vi "gums_measureLoopV3.vi"(0 "File Name":path=path "D:/users/test.dat", 1 "SaveDataQuery":bool=TRUE, 2 "Gain Cluster 2":T4={"Vsd"="Gate", "I 2probe 2"="Gate", "Vxy"="Gate", "Vxx"="Gate", "I leak BG"="Gate", "I leak TG"="Gate", "I Gain 1"=1000000.0, "V Gain 1"=1.0, "conversion factor BG"=1.0, "Vin / Vout 1"=1.0, "V Gain 2"=1.0, "Vin / Vout 2"=1.0, "V Gain 3"=1.0, "Vin / Vout 3"=1.0, "I Gain 2"=1000000.0, "I Gain 3"=1000000.0, "V BG"="Gate", "V TG"="Gate", "conversion factor TG"=1.0, "Vin / Vout 4"=1.0, "Vin / Vout 5"=1.0, "Manual Gain 1"=1.0, "Manual Gain 2"=1.0, "Manual Gain 3"=1.0, "V / I 4"="Gate", "V / I 3"="Gate", "Gain V/I3"=1.0, "Gain V/I4"=1.0} {"conversion factor TG" items=["1 V/V"=1.0, "4 V/V"=4.0, "15 V/V"=15.0, "30 V/V"=30.0, "45 V/V"=45.0]; "I Gain 3" items=["1"=1.0, "10"=10.0, "100"=100.0, "1K"=1000.0, "10K"=10000.0, "100K"=100000.0, "1M"=1000000.0, "10M"=10000000.0, "100M"=100000000.0, "1G"=1000000000.0]; "I Gain 2" items=["1"=1.0, "10"=10.0, "100"=100.0, "1K"=1000.0, "10K"=10000.0, "100K"=100000.0, "1M"=1000000.0, "10M"=10000000.0, "100M"=100000000.0, "1G"=1000000000.0]; "V Gain 3" items=["1"=1.0, "10"=10.0, "100"=100.0, "1K"=1000.0, "10K"=10000.0]; "V Gain 2" items=["1"=1.0, "10"=10.0, "100"=100.0, "1K"=1000.0, "10K"=10000.0]; "conversion factor BG" items=["1 V/V"=1.0, "4 V/V"=4.0, "15 V/V"=15.0, "30 V/V"=30.0, "45 V/V"=45.0]; "V Gain 1" items=["1"=1.0, "10"=10.0, "100"=100.0, "1K"=1000.0, "10K"=10000.0]; "I Gain 1" items=["1"=1.0, "10"=10.0, "100"=100.0, "1K"=1000.0, "10K"=10000.0, "100K"=100000.0, "1M"=1000000.0, "10M"=10000000.0, "100M"=100000000.0, "1G"=1000000000.0]}, 3 "Refresh Rate [ms]":i32=1000 min=0, 4 "Device Cluster":T5={"K2400 1"="", "K2400_1"=FALSE, "K2400 2"="", "K2400_2"=FALSE, "TIC"="", "Tcontrol"="OFF", "DAC"="", "DAC present"=FALSE, "Bfield query"=FALSE, "Wvlen query"=FALSE, "ITC signal"={"ITC"=0, "Signal"=enum."Sensor 1"}, "DMMX"=[["DMM1", ""]], "LockinX"=[["DMM1", ""]]}) -> ()   [LabVIEW 2011]
uses:
  Kelvinox drivers/ITCAPPS - Copie.LLB/ITCSignal.ctl
  Kelvinox drivers/ITCAPPS.LLB/ITCSignals.ctl
  Kelvinox drivers/BUSGEN.LLB/OxfordAddress.ctl
  stopButton.vi
  DAC/DACreadglobal.vi
  GlobalVar.vi
  monochromatorcontrol/perHandlemonochromator.vi
  Tglobalvar.vi
  monochromatorcontrol/libPhyspec.lvlib
panel:
  out "*(type *) &x":refnum<visa-resource-name>
  out "V/I4 array":dbl[](array[numeric])
  out "V/I3 array":dbl[](array[numeric])
  out "SetInstrument Cluster":cluster{dbl, dbl, dbl, dbl[], dbl, dbl, dbl}
  out "Lockin A all (V)":dbl[](array[numeric])
  out "Lockin A Array":dbl[][](array[numeric])
  out "signal cluster":T1
  out "Lockin Y all (V)":dbl[](array[numeric])
  out "Lockin X all (V)":dbl[](array[numeric])
  out "Lockin Y Array":dbl[][](array[numeric])
  out "Lockin X Array":dbl[][](array[numeric])
  out "LockinX":string[][](array[string])
  out "refnum raw":refnum<file>
  out "DMM all (V)":dbl[](array[numeric])
  out "DMM Array":dbl[][](array[numeric])
  out "DMMX":string[][](array[string])
  out "DAC 2 V [V]":dbl=1916.0
  out "DAC 2 array":dbl[](array[numeric])
  out "Formula4Array":dbl[](array[numeric]) format="%.2f"
  out "Formula3Array":dbl[](array[numeric]) format="%.2f"
  out "Formula2Array":dbl[](array[numeric]) format="%.2f"
  in  "Formula 4":string
  in  "Formula 3":string
  in  "Formula 2":string
  out "Formula1Array":dbl[](array[numeric]) format="%.2f"
  in  "Formula 1":string
  out "Rxy Array":dbl[](array[numeric])
  out "ITC signal":T2={"ITC"=0, "Signal"=enum."Sensor 1"}
  in  "Fig4 Y scale":string(combo)="0"
  in  "Y-Axis 4":string(combo)="Gate"
  in  "X-Axis 4":string(combo)="Gate"
  out "Isd 4":cluster{"Bg":dbl[], "V_4probe":dbl[]}(graph)
  in  "Fig3 Y scale":string(combo)="0"
  in  "Y-Axis 3":string(combo)="Gate"
  in  "X-Axis 3":string(combo)="Gate"
  in  "Fig1 Y scale":string(combo)="0"
  in  "Fig2 Y scale":string(combo)="0"
  out "Fig 2":cluster{"Bg":dbl[], "V_4probe":dbl[]}(graph)
  in  "Y-Axis 1":string(combo)="Gate"
  in  "X-Axis 1":string(combo)="Gate"
  out "R4probe array":dbl[](array[numeric])
  out "R2probe array":dbl[](array[numeric])
  out "Itg array":dbl[](array[numeric])
  out "Ibg array":dbl[](array[numeric])
  out "Vxy array":dbl[](array[numeric])
  out "Vxx array":dbl[](array[numeric])
  out "Isd array":dbl[](array[numeric])
  out "Vsd array":dbl[](array[numeric])
  out "Vtg array":dbl[](array[numeric])
  out "Vbg array":dbl[](array[numeric])
  out "R 4probe [kOhm]":dbl=1916.0
  out "V_topgate [V]":dbl=1916.0
  out "V_backgate [V]":dbl=1916.0
  out "Vxy [V]":dbl=1916.0
  out "Vxx [V]":dbl=1916.0
  out "R 2probe [kOhm]":dbl=1916.0
  out "I Leak TG[nA]":dbl=1916.0
  out "I Leak BG [nA]":dbl=1916.0
  out "I 2probe [nA]":dbl=1916.0
  out "Vsd [V]":dbl=1916.0
  in  "Sensitivity Lockin2":T6(ring)
  in  "Sensitivity Lockin1":T6(ring)
  out "Wavelength array":dbl[](array[numeric])
  out "Wavelength [nm]":dbl=1916.0
  out "Wvlen query":bool
  out "refnum data":refnum<file>
  in  "Y-Axis 2":string(combo)="Gate"
  in  "X-Axis 2":string(combo)="Gate"
  out "I K2400 01":dbl[](array[numeric])
  out "I K2400 02":dbl[](array[numeric])
  out "DAC 4 array":dbl[](array[numeric])
  out "DAC 3 array":dbl[](array[numeric])
  out "B":dbl[](array[numeric])
  out "B [T]":dbl=1916.0
  out "T [K]":dbl=1916.0
  out "Bfield query":bool
  out "I K2400_2 [A]":dbl=1916.0
  out "V / I 4 [V or A]":dbl=1916.0
  out "V / I 3 [V or A]":dbl=1916.0
  out "DAC 4 V [V]":dbl=1916.0
  out "DAC 3 V [V]":dbl=1916.0
  out "I K2400_1 [A]":dbl=1916.0
  out "Lockin1 Y [V]":dbl=1916.0
  out "Lockin1 X [V]":dbl=1916.0
  out "Lockin1 Ampl [V]":dbl=1916.0
  out "K2400 1 [V]":dbl=1916.0
  out "K2400 2 [V]":dbl=1916.0
  out "DAC 1 V [V]":dbl=1916.0
  out "DAC present":bool
  out "K2400_2":bool
  out "K2400 2":refnum<visa-resource-name>="GPIB0::11::INSTR"
  out "DAC":refnum<visa-resource-name>="GPIB0::11::INSTR"
  out "Tcontrol":string
  out "K2400_1":bool
  out "TIC":refnum<visa-resource-name>="GPIB0::11::INSTR"
  out "K2400 1":refnum<visa-resource-name>="GPIB0::11::INSTR"
  out "Isd":cluster{"Bg":dbl[], "V_4probe":dbl[]}(graph)
  out "Isd 3":cluster{"Bg":dbl[], "V_4probe":dbl[]}(graph)
  out "stopMainLoop":bool
  out "V K2400_01 array":dbl[](array[numeric])
  out "DAC 1 array":dbl[](array[numeric])
  out "V K2400_02 array":dbl[](array[numeric])
  out "T":dbl[](array[numeric])
  out "Time":dbl[](array[numeric])
  out "Time [s]":dbl=1916.0
  in  "stop":bool
  # "Current run values"
  # "Magnetic Field"
  # "Wavelength"
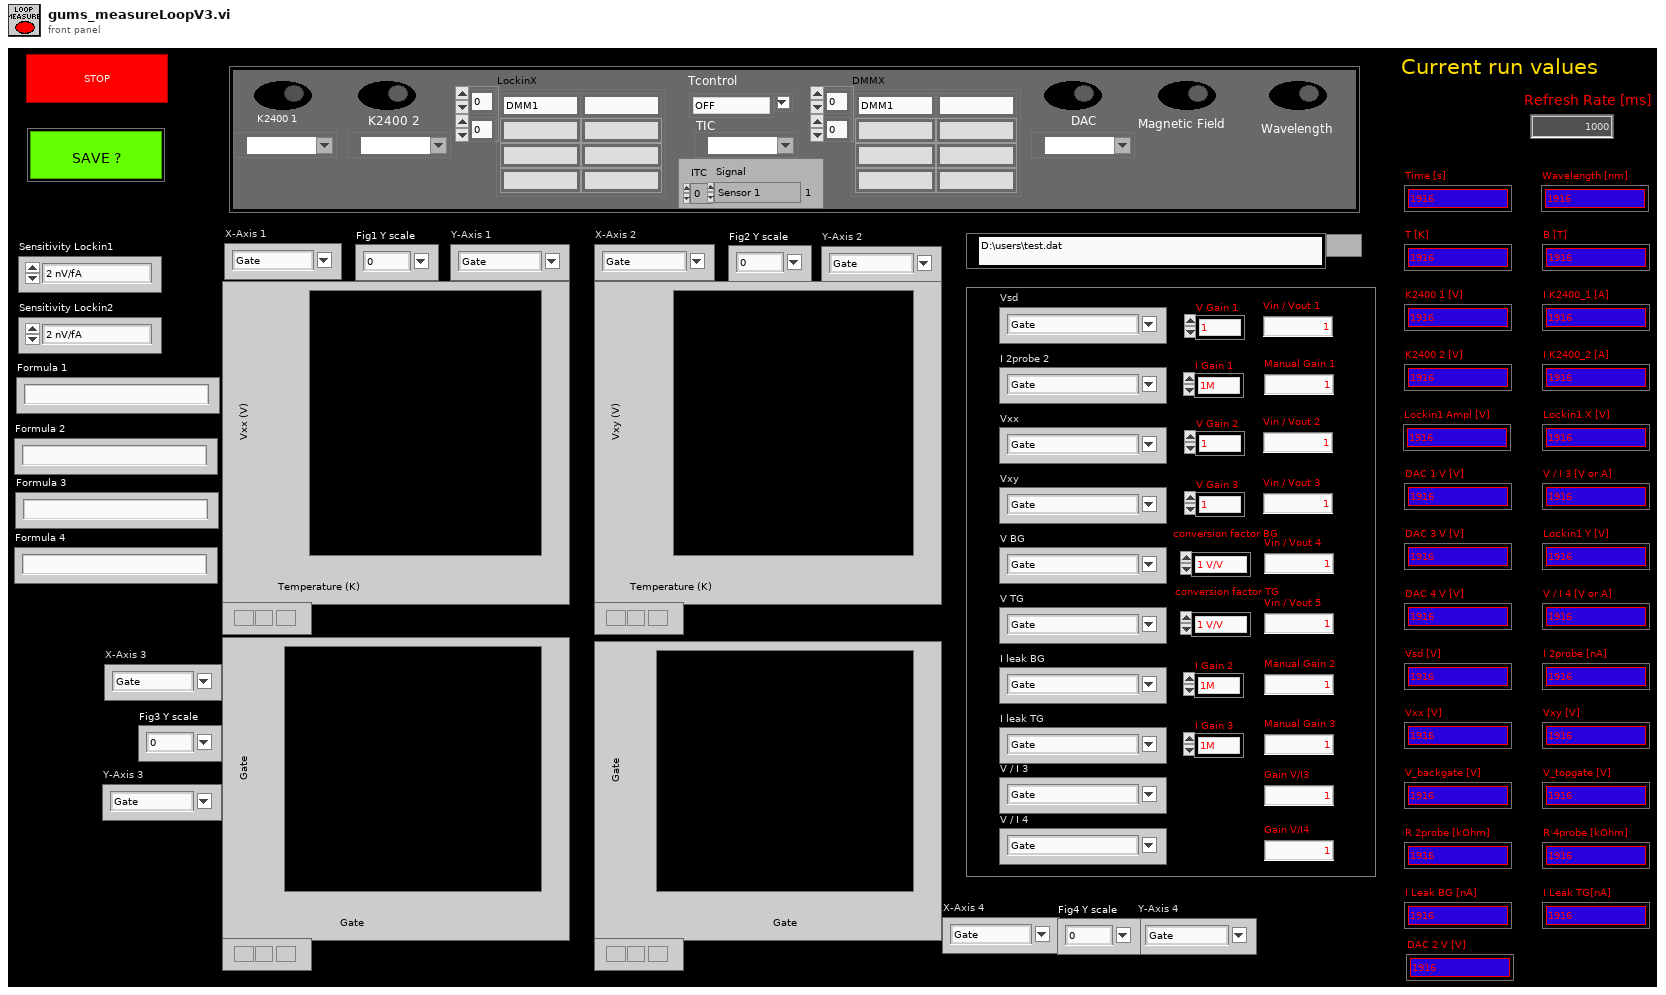
[diagram p1: front panel]
types:
  T1 = cluster{dbl[], dbl[], "I K2400_1 [A]":dbl, "I K2400_2 [A]":dbl, dbl[]}
  T2 = typedef "ITCSignal.ctl" = cluster{"ITC":u16, "Signal":T3}
  T3 = typedef "ITCSignals.ctl" = enum16{"Setpoint", "Sensor 1", "Sensor 2", "Sensor 3", "Needle Valve %", "Heater %"}
  T4 = cluster{"Vsd":string, "I 2probe 2":string, "Vxy":string, "Vxx":string, "I leak BG":string, "I leak TG":string, "I Gain 1":dbl, "V Gain 1":dbl, "conversion factor BG":dbl, "Vin / Vout 1":dbl, "V Gain 2":dbl, "Vin / Vout 2":dbl, "V Gain 3":dbl, "Vin / Vout 3":dbl, "I Gain 2":dbl, "I Gain 3":dbl, "V BG":string, "V TG":string, "conversion factor TG":dbl, "Vin / Vout 4":dbl, "Vin / Vout 5":dbl, "Manual Gain 1":dbl, "Manual Gain 2":dbl, "Manual Gain 3":dbl, "V / I 4":string, "V / I 3":string, "Gain V/I3":dbl, "Gain V/I4":dbl}
  T5 = cluster{"K2400 1":refnum<visa-resource-name>, "K2400_1":bool, "K2400 2":refnum<visa-resource-name>, "K2400_2":bool, "TIC":refnum<visa-resource-name>, "Tcontrol":string, "DAC":refnum<visa-resource-name>, "DAC present":bool, "Bfield query":bool, "Wvlen query":bool, "ITC signal":T2, "DMMX":string[][], "LockinX":string[][]}
  T6 = enum16{"2 nV/fA", "5 nV/fA", "10 nV/fA", "20 nV/fA", "50 nV/fA", "100 nV/fA", "200 nV/fA", "500 nV/fA", "1 uV/pA", "2 uV/pA", "5 uV/pA", "10 uV/pA", "20 uV/pA", "50 uV/pA", "100 uV/pA", "200 uV/pA", "500 uV/pA", "1 mV/nA", "2 mV/nA", "5 mV/nA", "10 mV/nA", "20 mV/nA", "50 mV/nA", "100 mV/nA", "200 mV/nA", "500 mV/nA", "1 V/uA"}
  T7 = typedef "OxfordAddress.ctl" = cluster{"Com Port":i32, "ISOBUS Address":i32, "GPIB Address":i16, "Communication":enum16{"RS232", "ISOBUS", "GPIB", "Gateway"}}
  T8 = enum16{"open", "replace", "create", "open or create", "replace or create", "replace or create with confirmation"}
  T9 = cluster{"Formula4Array":dbl[], "Formula4Array":dbl[]}
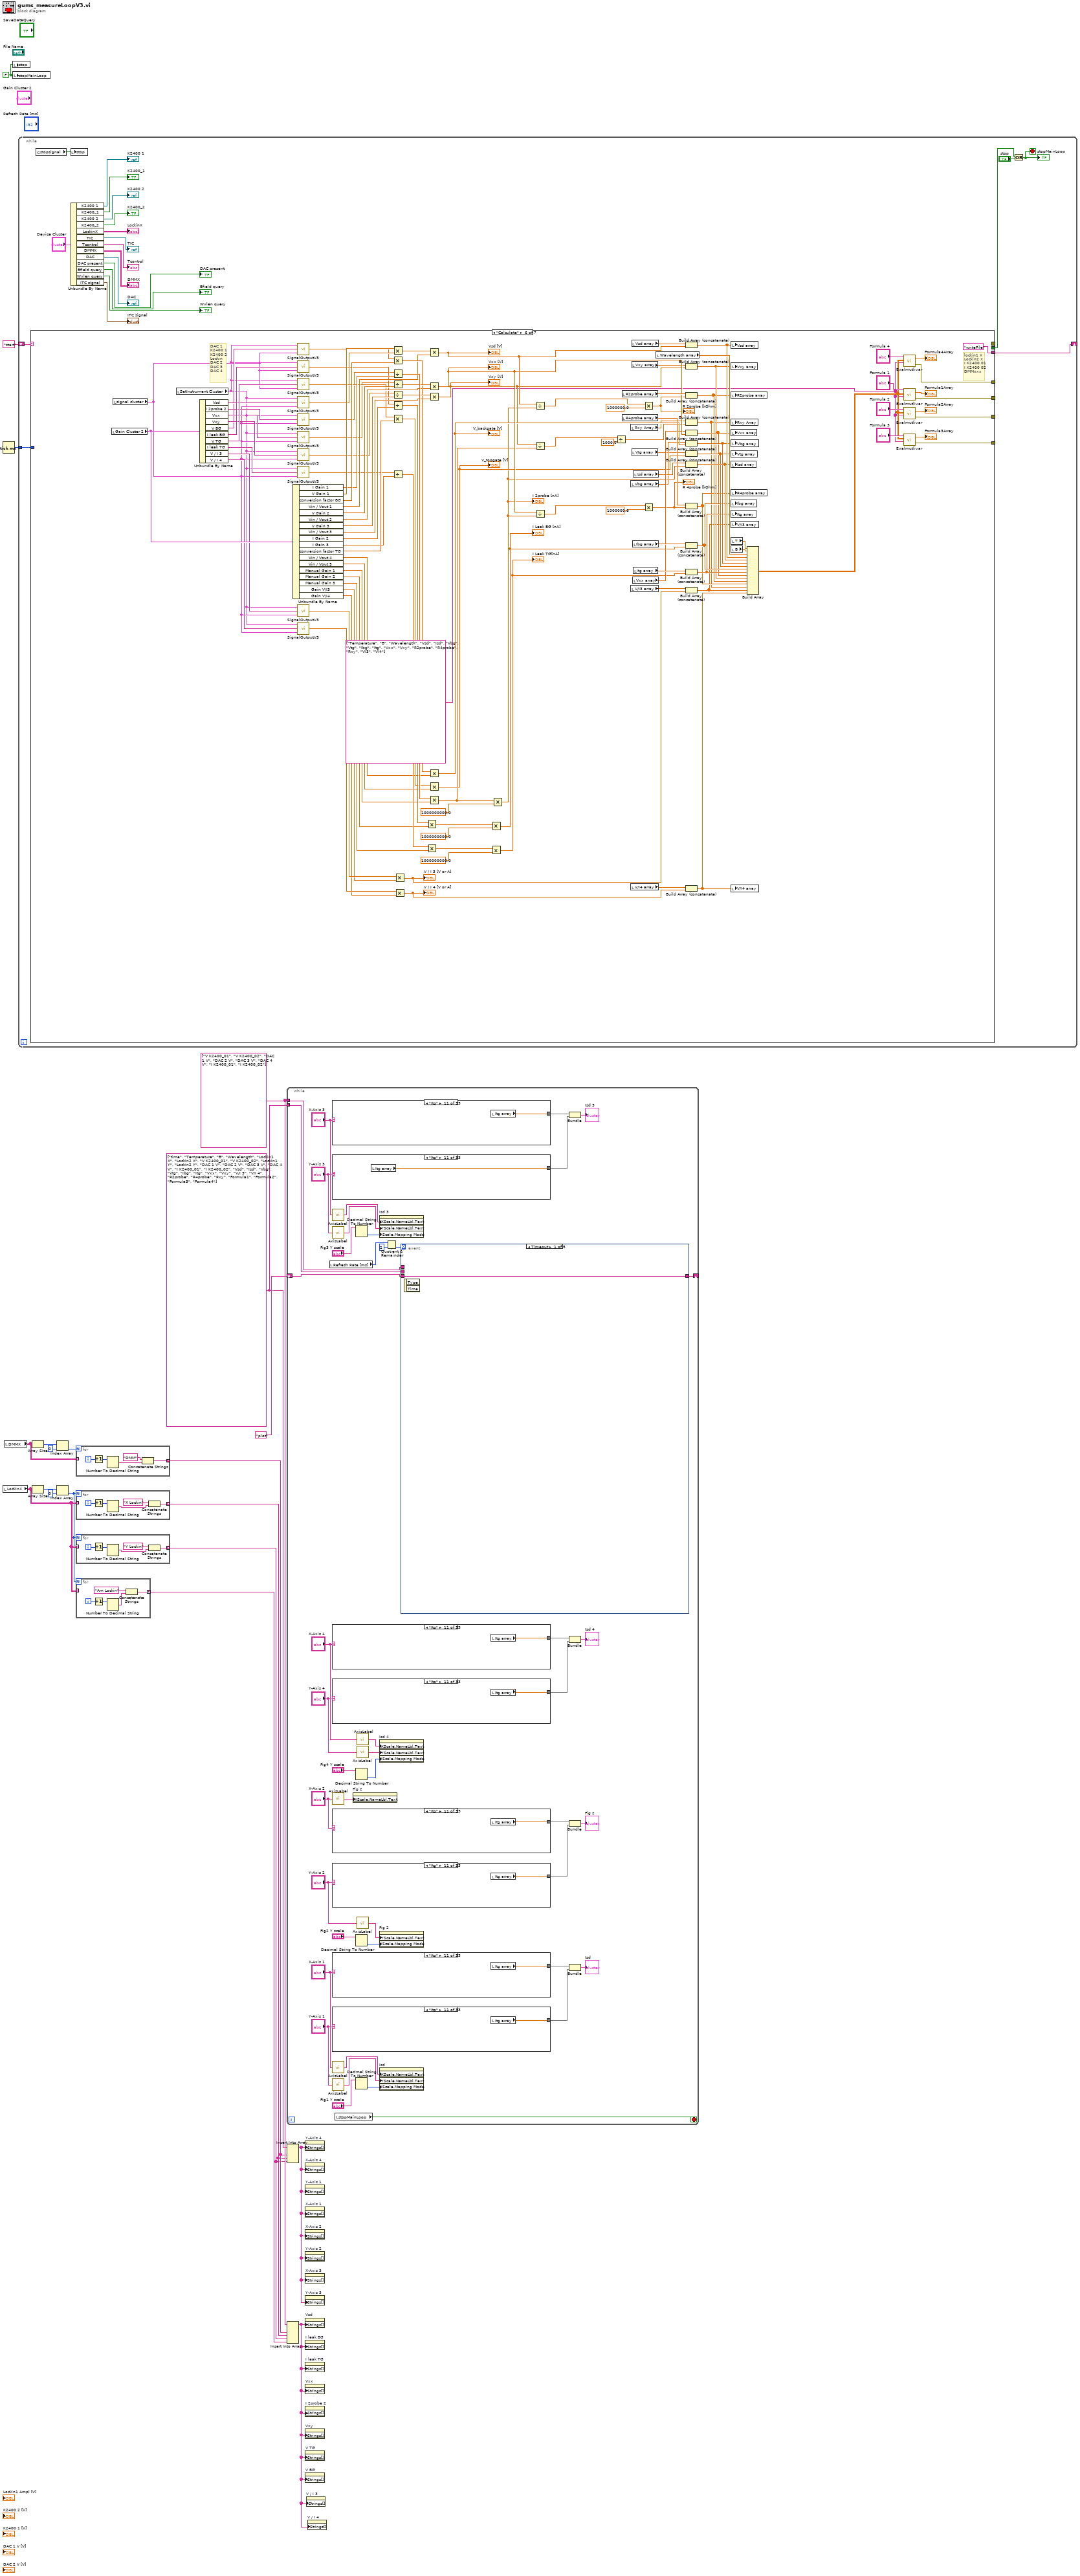
[diagram p0: block diagram]
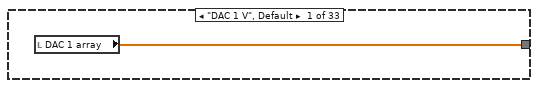
[diagram p2: hidden frame]
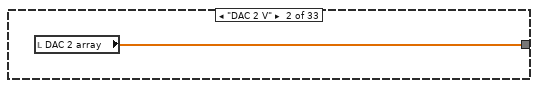
[diagram p3: hidden frame]
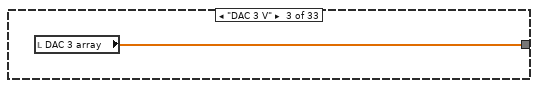
[diagram p4: hidden frame]
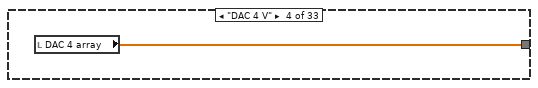
[diagram p5: hidden frame]
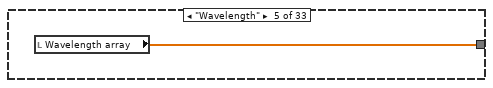
[diagram p6: hidden frame]
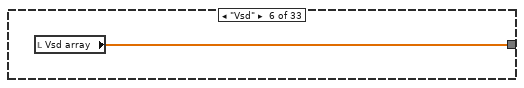
[diagram p7: hidden frame]
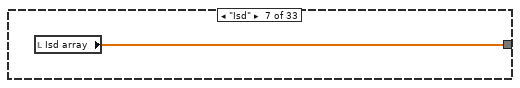
[diagram p8: hidden frame]
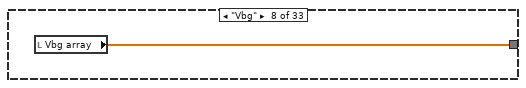
[diagram p9: hidden frame]
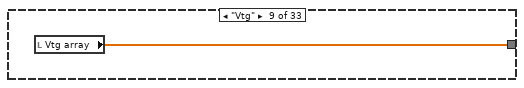
[diagram p10: hidden frame]
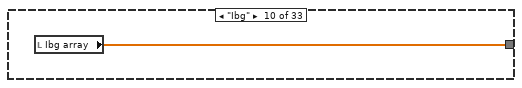
[diagram p11: hidden frame]
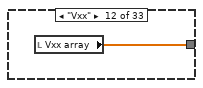
[diagram p12: hidden frame]
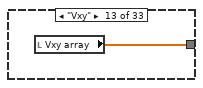
[diagram p13: hidden frame]
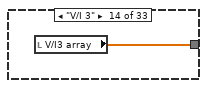
[diagram p14: hidden frame]
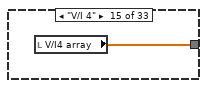
[diagram p15: hidden frame]
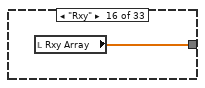
[diagram p16: hidden frame]
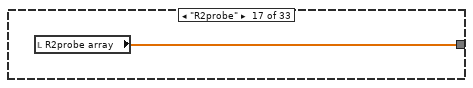
[diagram p17: hidden frame]
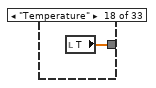
[diagram p18: hidden frame]
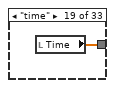
[diagram p19: hidden frame]
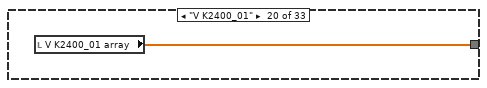
[diagram p20: hidden frame]
diagram:
  w10 = string[] ["time", "Temperature", "B", "Wavelength", "Lockin1 X", "Lockin2 X", "V K2400_01", "V K2400_02", "Lockin1 Y", "Lockin2 Y", "DAC 1 V", "DAC 2 V", "DAC 3 V", "DAC 4 V", "I K2400_01", "I K2400_02", "Vsd", "Isd", "Vbg", "Vtg", "Ibg", "Itg", "Vxx", "Vxy", "V/I 3", "V/I 4", "R2probe", "R4probe", "Rxy", "Formula1", "Formula2", "Formula3", "Formula4"] ("Axis select")
  w9 = string[] ["V K2400_01", "V K2400_02", "DAC 1 V", "DAC 2 V", "DAC 3 V", "DAC 4 V", "I K2400_01", "I K2400_02"] ("Strings []")
  w18 = FALSE ("stop")
  n1 = Tick Count (ms)() -> (millisecond timer value=w19:u32)
  n2 = local read "LockinX"() -> (w4:string[][])
  n3 = local read "DMMX"() -> (w14:string[][])
  n4 = local write "stop"(w18) -> ()
  n5 = local write "stopMainLoop"(w18) -> ()
  n6 = while {
    shift-right: [w40] -> _
    shift-left: "start" -> [w41]
    tunnel: w19 -> [w37]
    stop <- w36 stop-if-true
    n7 = case shown="\"Calculate\"" w41 {
      tunnel: ["measureSetInstruments" "measureSignal" "measureOutParam" "Calculate" "measureSetInstruments" "writeFile" ""] -> w40
      tunnel: [_ _ _ _ _ _ TRUE ("x")] -> w38
      tunnel: w37 -> [_ _ _ w343 _ _ _]
      tunnel: [_ _ _ _ w370 _ _] -> _
      tunnel: [_ _ _ _ _ w511 _] -> _
      tunnel: [_ _ _ _ _ w501 _] -> _
      tunnel: [_ _ _ _ _ w500 _] -> _
      tunnel: [_ _ _ _ _ w499 _] -> _
      frame "start", Default {
        w43 = "\t"
        w62 = enum16{"start", "end", "current"}."end" ("from (0:start)")
        w67 = T8."open or create" ("operation (0:open)")
        w93 = 0 ("dimension size")
        w42 = "\t"
        w102 = "\t"
        w110 = "\t"
        w77 = "\t"
        w114 = "\t"
        w111 = "\t"
        (unwired) "Lockin1 X [V]" ("string")
        w117 = "\t"
        # "Time\nT\nB\nWavelength\nDAC1\nDAC2\nDAC3\nDAC4\nV K2400_01\nV K2400_02\nLockin V\nLK 1 X\nLK 1 Y\nLK2 X\nLK2 Y\nDMMX\nI K2400_01\nI K2400_02\n\nTime\nT\nB\nWavelength\nVsd\nVbgate\nVtopgate\nI2probe\nIleak bg\nIleak tg\nVxx\nVxy\nR2probe\nR4probe"
        n8 = Get Date/Time In Seconds() -> (seconds since 1Jan1904=w128:timestamp)
        n9 = Initialize Array(0) -> (→"Time" →"T" →"DAC 1 array" →"V K2400_01 array" →"V K2400_02 array" →"B" →"DAC 3 array" →"DAC 4 array" →"I K2400 02" →"I K2400 01" →"Wavelength array" →"Vbg array" →"Vtg array" →"Vsd array" →"Isd array" →"Vxx array" →"Vxy array" →"Ibg array" →"Itg array" →"R2probe array" →"R4probe array" →"Rxy Array" →"DAC 2 array" →"V/I3 array" →"V/I4 array":i32[])  [unwired: 1 out]
        n10 = Initialize Array(w93, w93, w93) -> (→"DMM Array" →"Lockin X Array" →"Lockin Y Array" →"Lockin A Array":i32[][])
        n11 = local read "File Name"() -> (w87:path)
        n12 = local read "LockinX"() -> (w55:string[][])
        n13 = local read "DMMX"() -> (w70:string[][])
        n14 = Get Date/Time String(date format (0)=1, seconds (now)=w128) -> (date string=w125:string, time string=w126:string)  [unwired: 1 out]
        n15 = Array Size(array=w55) -> (size(s)=w56:i32[])
        n16 = Array Size(array=w70) -> (size(s)=w73:i32[])
        n17 = Strip Path(path=w87) -> (stripped path=w92:path, name=w91:string)
        n18 = Open/Create/Replace File(file path (use dialog)=w87, prompt="Enter data filename", operation (0:open)=w67) -> (refnum out=w66:refnum<file>, error out=w65:errorcluster)  [unwired: 1 in, 3 out]
        n19 = Concatenate Strings(w126, "\t", w125, "\r\n") -> (w81:string)
        n20 = Index Array(array=w73, index=0) -> (element=w72:i32)
        n21 = Index Array(array=w56, index=0) -> (element=w53:i32)
        n22 = for {
          N: w53 -> [_]
          tunnel: [w134] -> w52 mode=indexing
          i -> [w137]
          n23 = Increment(x=w137) -> (x+1=w135:i32)
          n24 = Number To Decimal String(number=w135) -> (decimal integer string=w136:string)  [unwired: 1 in]
          n25 = Concatenate Strings("Lockin", w136, " A [V]" ("string"), "\t") -> (w134:string)
        }
        n26 = for {
          N: w53 -> [_]
          tunnel: [w148] -> w51 mode=indexing
          i -> [w151]
          n27 = Increment(x=w151) -> (x+1=w149:i32)
          n28 = Number To Decimal String(number=w149) -> (decimal integer string=w150:string)  [unwired: 1 in]
          n29 = Concatenate Strings("Lockin", w150, " X [V]" ("string"), "\t") -> (w148:string)
        }
        n30 = for {
          N: w53 -> [_]
          tunnel: [w141] -> w50 mode=indexing
          i -> [w144]
          n31 = Increment(x=w144) -> (x+1=w142:i32)
          n32 = Number To Decimal String(number=w142) -> (decimal integer string=w143:string)  [unwired: 1 in]
          n33 = Concatenate Strings("Lockin", w143, " Y [V]" ("string"), "\t") -> (w141:string)
        }
        n34 = for {
          N: w72 -> [_]
          tunnel: [w155] -> w69 mode=indexing
          i -> [w158]
          n35 = Increment(x=w158) -> (x+1=w156:i32)
          n36 = Number To Decimal String(number=w156) -> (decimal integer string=w157:string)  [unwired: 1 in]
          n37 = Concatenate Strings("DMM", w157, " [V]" ("string"), "\t") -> (w155:string)
        }
        n38 = Concatenate Strings("Vxx [V]" ("string"), w42, "Vxy [V]" ("string"), w42, "R2probe [kOhm]" ("string"), w42, "R4probe [kOhm]" ("string"), w42) -> (w96:string)
        n39 = Concatenate Strings("I 2probe [nA]" ("string"), w102, "Ileak bg [nA]" ("string"), w102, "Ileak tg [nA]" ("string"), w102) -> (w101:string)
        n40 = Concatenate Strings("Vsd [V]" ("string"), w110, "Vbg [V]" ("string"), w110, "Vtg [V]" ("string"), w110) -> (w106:string)
        n41 = Concatenate Strings("Time [s]", w117, "T [K]" ("chaîne"), w117, "B [T]" ("chaîne"), w117, "Wavelength [nm]" ("chaîne"), w117) -> (w78:string)
        n42 = Concatenate Strings("V/I3 [V or A]" ("string"), w43, "V/I4 [V or A]" ("string"), w43) -> (w46:string)
        n43 = Search and Replace String(input string=w91, search string=".dat", replace string="_raw.dat" ("replace string (\"\")")) -> (result string=w88:string)  [unwired: 5 in, 3 out]
        n44 = Set File Position(refnum=w66, from (0:start)=w62, error in=w65) -> (refnum out=w63:refnum<file>, error out=w64:errorcluster)  [unwired: 1 in]
        n45 = Build Path(base path=w92, name or relative path=w88) -> (appended path=w86:path)
        n46 = Concatenate Strings(w81, w78, w106, w101, w96, w46, "\r\n") -> (w122:string)
        n47 = Write to Text File(file (use dialog)=w63, text=w122, error in=w64) -> (refnum out=→"refnum data":refnum<file>, error out=w85:errorcluster)  [unwired: 2 out]
        n48 = Concatenate Strings("DAC 1 [V]" ("string"), w77, "DAC 2 [V]" ("string"), w77, "DAC 3 [V]" ("string"), w77, "DAC 4 [V]" ("string"), w77, "K2400_01 [V]" ("string"), w77, "K2400_02 [V]" ("string"), w77, w52, w77) -> (w79:string)
        n49 = Concatenate Strings(w51, w114, w50, w114) -> (w80:string)
        n50 = Concatenate Strings("I K2400_01 [A]" ("string"), w111, "I K2400_02 [A]" ("string"), w111) -> (w71:string)
        n51 = Open/Create/Replace File(file path (use dialog)=w86, error in=w85, operation (0:open)=w67) -> (refnum out=w59:refnum<file>, error out=w61:errorcluster)  [unwired: 1 in, 3 out]
        n52 = Concatenate Strings(w81, w78, w79, w80, w69, w71, "\r\n") -> (w68:string)
        n53 = Set File Position(refnum=w59, from (0:start)=w62, error in=w61) -> (refnum out=w58:refnum<file>, error out=w60:errorcluster)  [unwired: 1 in]
        n54 = Write to Text File(file (use dialog)=w58, text=w68, error in=w60) -> (refnum out=→"refnum raw":refnum<file>, error out=w83:errorcluster)  [unwired: 2 out]
        n55 = case shown="No Error" w83 {
          frame No Error {
          }
          frame Error {
          }
        }
      }
      frame "measureSetInstruments" {
        w186 = errorcluster {"status"=FALSE, "code"=0, "source"=""} ("error in (no error)")
        w160 = 0.0
        # "DAC 1\nK2400 1\nK2400 2\nLockin\nDAC 2\nDAC 3\nDAC 4"
        n56 = local read "K2400_1"() -> (w200:bool)
        n57 = local read "K2400_2"() -> (w199:bool)
        n58 = local read "LockinX"() -> (w168:string[][])
        n59 = local read "K2400 1"() -> (w192:refnum<visa-resource-name>)
        n60 = local read "K2400 2"() -> (w191:refnum<visa-resource-name>)
        n61 = case shown="True" w200 {
          tunnel: [w257 w262] -> w189
          tunnel: w160 -> [w257 _]
          tunnel: w192 -> [_ w261]
          tunnel: w186 -> [_ _]
          tunnel: [w257 w258] -> w185
          frame False {
          }
          frame True {
            n62 = call "K2400_write&read.vi"("Command"="READ?", "VISA Resource Name"=w261) -> ("error out"=w260:errorcluster, "Read"=w266:string)  [unwired: 1 in]
            n63 = case shown="No Error" w260 {
              frame No Error {
              }
              frame Error {
              }
            }
            n64 = Match Pattern(string=w266, regular expression=",") -> (before substring=w263:string, after substring=w259:string)  [unwired: 3 out]
            n65 = Fract/Exp String To Number(string=w263) -> (number=w262:dbl)  [unwired: 4 out]
            n66 = Fract/Exp String To Number(string=w259) -> (number=w258:dbl)  [unwired: 4 out]
          }
        }
        "I K2400_1 [A]" <- w185
        n67 = case shown="True" w199 {
          tunnel: [w246 w252] -> w188
          tunnel: w160 -> [w246 _]
          tunnel: w191 -> [_ w251]
          tunnel: w186 -> [_ w250]
          tunnel: [w246 w247] -> w184
          frame False {
          }
          frame True {
            n68 = call "K2400_write&read.vi"("error in (no error)"=w250, "Command"="READ?", "VISA Resource Name"=w251) -> ("error out"=w249:errorcluster, "Read"=w256:string)
            n69 = case shown="No Error" w249 {
              frame No Error {
              }
              frame Error {
              }
            }
            n70 = Match Pattern(string=w256, regular expression=",") -> (before substring=w253:string, after substring=w248:string)  [unwired: 3 out]
            n71 = Fract/Exp String To Number(string=w253) -> (number=w252:dbl)  [unwired: 4 out]
            n72 = Fract/Exp String To Number(string=w248) -> (number=w247:dbl)  [unwired: 4 out]
          }
        }
        "I K2400_2 [A]" <- w184
        n73 = Array Size(array=w168) -> (size(s)=w170:i32[])
        n74 = local read "Wvlen query"() -> (w164:bool)
        n75 = global read "DACreadglobal.vi" "DAC read global (mV)"() -> (w179:dbl[])
        n76 = case shown="True" w164 {
          tunnel: w160 -> [w202 _]
          tunnel: [w202 w207] -> w162
          tunnel: [_ w206] -> _
          frame False {
          }
          frame True {
            n77 = global read "GlobalVar.vi" "Stabilizing"() -> (w205:bool)
            n78 = global read "perHandlemonochromator.vi" "peHandle"() -> (w204:u32)
            n79 = case shown="True" w205 {
              tunnel: w204 -> [w208 w211]
              tunnel: [w208 w211] -> w203
              frame False {
                n80 = while {
                  stop <- w210 stop-if-true
                  n81 = global read "GlobalVar.vi" "Stabilizing"() -> (w210:bool)
                  n82 = Wait (ms)(milliseconds to wait=u32 5) -> ()  [unwired: 1 out]
                }
              }
              frame True {
              }
            }
            n83 = call "PE Get Wavelength.vi"("peHandle"=w203) -> ("error out"=w206:errorcluster, "wavelength"=w207:dbl)  [unwired: 8 in, 1 out]
          }
        }
        "Wavelength [nm]" <- w162
        n84 = local read "DAC present"() -> (w180:bool)
        n85 = Index Array(array=w170, index=0) -> (element=w169:i32)
        n86 = for {
          N: w169 -> [_]
          tunnel: w168 -> [w224] mode=indexing
          tunnel: [w213] -> _ mode=indexing
          tunnel: [w212] -> w165 mode=indexing
          n87 = Index Array(array=w224, index=1) -> (element=w220:string)
          n88 = Concatenate Strings("GPIB0::" ("string"), w220) -> (w219:string)
          n89 = Type Cast(type=refnum<visa-resource-name> refnum ("VISA resource name"), x=w219) -> (*(type *) &x=w213:refnum<visa-resource-name>)
          "*(type *) &x" <- w213
          n90 = VISA Write(VISA resource name=w213, write buffer="SLVL? " ("chaîne")) -> (VISA resource name out=w217:refnum<visa-resource-name>, error out=w216:errorcluster)  [unwired: 1 in, 1 out]
          n91 = VISA Read(VISA resource name=w217, byte count=u32 1024, error in (no error)=w216) -> (read buffer=w214:string)  [unwired: 3 out]
          n92 = Fract/Exp String To Number(string=w214) -> (number=w212:dbl)  [unwired: 4 out]
        }
        "Lockin A all (V)" <- w165
        n93 = local read "DAC"() -> (w183:refnum<visa-resource-name>)
        n94 = case shown="True" w180 {
          selector: w180 -> [w227 w243]
          tunnel: [w225 w244] -> w190
          tunnel: w160 -> [w225 _]
          tunnel: w183 -> [_ _]
          tunnel: [w227 w243] -> _
          tunnel: w179 -> [w226 w230]
          tunnel: [w226 w230] -> _
          tunnel: [w225 w237] -> w178
          tunnel: [w225 w229] -> w173
          tunnel: [w225 w228] -> w172
          frame False {
          }
          frame True {
            # "dac 4"
            # "dac 3"
            n95 = Index Array(array=w230, index=0) -> (element=w241:dbl)
            n96 = Index Array(array=w230, index=1) -> (element=w240:dbl)
            n97 = Index Array(array=w230, index=2) -> (element=w236:dbl)
            n98 = Index Array(array=w230, index=3) -> (element=w233:dbl)
            n99 = Divide(x=w241, y=1000.0) -> (x/y=w244:dbl)
            n100 = Divide(x=w240, y=1000.0) -> (x/y=w237:dbl)
            n101 = Divide(x=w236, y=1000.0) -> (x/y=w229:dbl)
            n102 = Divide(x=w233, y=1000.0) -> (x/y=w228:dbl)
          }
        }
        "DAC 3 V [V]" <- w173
        "DAC 4 V [V]" <- w172
        n103 = local read "Wavelength array"() -> (w163:dbl[])
        n104 = Build Array (concatenate)(w163, w162) -> (w161:dbl[])
        n105 = local read "DAC 4 array"() -> (w175:dbl[])
        n106 = local read "DAC 2 array"() -> (w182:dbl[])
        n107 = local read "DAC 1 array"() -> (w198:dbl[])
        n108 = local read "DAC 3 array"() -> (w177:dbl[])
        n109 = local write "Wavelength array"(w161) -> ()
        n110 = local read "V K2400_01 array"() -> (w195:dbl[])
        n111 = local read "V K2400_02 array"() -> (w196:dbl[])
        n112 = local write "DAC 1 V [V]"(w190) -> ()
        n113 = local write "DAC 2 V [V]"(w178) -> ()
        n114 = Build Array (concatenate)(w175, w172) -> (w174:dbl[])
        n115 = Build Array (concatenate)(w182, w178) -> (w181:dbl[])
        n116 = Build Array (concatenate)(w198, w190) -> (w197:dbl[])
        n117 = Build Array (concatenate)(w177, w173) -> (w176:dbl[])
        n118 = local write "DAC 4 array"(w174) -> ()
        n119 = local write "K2400 1 [V]"(w189) -> ()
        n120 = local write "DAC 2 array"(w181) -> ()
        n121 = local write "DAC 1 array"(w197) -> ()
        n122 = local write "DAC 3 array"(w176) -> ()
        n123 = local write "K2400 2 [V]"(w188) -> ()
        n124 = Build Array (concatenate)(w195, w189) -> (w193:dbl[])
        n125 = Build Array (concatenate)(w196, w188) -> (w194:dbl[])
        n126 = local write "V K2400_01 array"(w193) -> ()
        n127 = local write "V K2400_02 array"(w194) -> ()
        n128 = local read "Lockin A Array"() -> (w167:dbl[][])
        n129 = Bundle(w190, w189, w188, w165, w178, w173, w172) -> (→"SetInstrument Cluster":cluster{dbl, dbl, dbl, dbl[], dbl, dbl, dbl})  [unwired: 1 in]
        n130 = Build Array (concatenate)(w167, w165) -> (w166:dbl[][])
        n131 = local write "Lockin A Array"(w166) -> ()
      }
      frame "measureSignal" {
        w269 = 0 ("index")
        (unwired) "1,4" ("Variable")
        w297 = 0.0
        # "lockin1 X\nLockin2 X\nI K2400 01\nI K2400 02\nDMMxxx"
        n132 = local read "LockinX"() -> (w278:string[][])
        n133 = local read "K2400_1"() -> (w300:bool)
        n134 = local read "K2400 1"() -> (w301:refnum<visa-resource-name>)
        n135 = local read "DMMX"() -> (w286:string[][])
        n136 = Array Size(array=w278) -> (size(s)=w280:i32[])
        n137 = Array Size(array=w286) -> (size(s)=w288:i32[])
        n138 = case shown="False" w300 {
          tunnel: [w325 w326] -> w290
          tunnel: w301 -> [_ _]
          tunnel: w297 -> [w325 _]
          tunnel: "READ?" -> [w324 w327]
          tunnel: [w324 w327] -> w291
          frame False {
          }
          frame True {
            n139 = local read "I K2400_1 [A]"() -> (w326:dbl)
          }
        }
        n140 = Index Array(array=w280, index=0) -> (element=w279:i32)
        n141 = Index Array(array=w288, index=0) -> (element=w285:i32)
        n142 = for {
          N: w285 -> [_]
          tunnel: w286 -> [w321] mode=indexing
          tunnel: [w315] -> _ mode=indexing
          tunnel: [w314] -> w282 mode=indexing
          n143 = Index Array(array=w321, index=1) -> (element=w317:string)
          n144 = Concatenate Strings("GPIB0::" ("string"), w317) -> (w316:string)
          n145 = Type Cast(type=refnum<visa-resource-name> refnum ("VISA resource name"), x=w316) -> (*(type *) &x=w315:refnum<visa-resource-name>)
          n146 = call "AGILENT34401a_read.vi"("VISA Resource Name in"=w315) -> ("Voltage output"=w314:dbl, "error out"=w313:errorcluster)  [unwired: 1 out]
          n147 = case shown="No Error" w313 {
            frame No Error {
            }
            frame Error {
            }
          }
        }
        "DMM all (V)" <- w282
        n148 = for {
          N: w279 -> [_]
          tunnel: w278 -> [w312] mode=indexing
          tunnel: [w306] -> _ mode=indexing
          tunnel: [w303] -> w270 mode=indexing
          tunnel: "1,4" ("Variable") -> [w305]
          tunnel: [w304] -> w271 mode=indexing
          n149 = Index Array(array=w312, index=1) -> (element=w308:string)
          n150 = Concatenate Strings("GPIB0::" ("string"), w308) -> (w307:string)
          n151 = Type Cast(type=refnum<visa-resource-name> refnum ("VISA resource name"), x=w307) -> (*(type *) &x=w306:refnum<visa-resource-name>)
          n152 = call "Lockin_SR830_readXY.vi"("Variable"=w305, "VISA Resource Name"=w306) -> ("Output Y"=w303:dbl, "Output X"=w304:dbl)
        }
        "Lockin X all (V)" <- w271
        "Lockin Y all (V)" <- w270
        n153 = local read "I K2400 01"() -> (w296:dbl[])
        n154 = local read "K2400_2"() -> (w298:bool)
        n155 = local read "K2400 2"() -> (w299:refnum<visa-resource-name>)
        n156 = case shown="False" w298 {
          tunnel: [w322 w323] -> w289
          tunnel: w299 -> [_ _]
          tunnel: w297 -> [w322 _]
          tunnel: w291 -> [_ _]
          frame False {
          }
          frame True {
            n157 = local read "I K2400_2 [A]"() -> (w323:dbl)
          }
        }
        n158 = Build Array (concatenate)(w296, w290) -> (w295:dbl[])
        n159 = local write "I K2400 01"(w295) -> ()
        n160 = local read "I K2400 02"() -> (w293:dbl[])
        n161 = Build Array (concatenate)(w293, w289) -> (w294:dbl[])
        n162 = local read "Lockin X Array"() -> (w276:dbl[][])
        n163 = local read "Lockin Y Array"() -> (w275:dbl[][])
        n164 = local read "DMM Array"() -> (w284:dbl[][])
        n165 = local write "I K2400 02"(w294) -> ()
        n166 = Index Array(array=w271, index=w269) -> (element=→"Lockin1 X [V]":dbl)
        n167 = Index Array(array=w270, index=w269) -> (element=→"Lockin1 Y [V]":dbl)
        n168 = Build Array (concatenate)(w276, w271) -> (w274:dbl[][])
        n169 = Build Array (concatenate)(w275, w270) -> (w273:dbl[][])
        n170 = Bundle(w271, w270, "I K2400_1 [A]"=w290, "I K2400_2 [A]"=w289, w282) -> (→"signal cluster":T1)  [unwired: 1 in]
        n171 = Build Array (concatenate)(w284, w282) -> (w283:dbl[][])
        n172 = local write "Lockin X Array"(w274) -> ()
        n173 = local write "Lockin Y Array"(w273) -> ()
        n174 = local write "DMM Array"(w283) -> ()
      }
      frame "measureOutParam" {
        n175 = Tick Count (ms)() -> (millisecond timer value=w346:u32)
        n176 = local read "Bfield query"() -> (w341:bool)
        n177 = Subtract(x=w346, y=w343) -> (x-y=w344:u32)
        n178 = local read "Tcontrol"() -> (w342:string)
        n179 = case shown="True" w341 {
          tunnel: [w348 w349] -> w335
          tunnel: 0.0 -> [w348 _]
          frame False {
          }
          frame True {
            n180 = call "TeslReadField.vi"() -> ("Effective field"=w350:dbl[unit])  [unwired: 6 in, 1 out]
            n181 = node(w350) -> (w349:dbl)
          }
        }
        "B [T]" <- w335
        n182 = local read "TIC"() -> (w334:refnum<visa-resource-name>)
        n183 = Quotient & Remainder(x=w344, y=u32 10) -> (floor(x/y)=w330:u32)  [unwired: 1 out]
        n184 = case shown="\"GlobalVar\"" w342 {
          tunnel: [0.0 w353 w357 w359 w368] -> w338
          tunnel: w334 -> [_ w352 _ _ _]
          frame "OFF", Default {
          }
          frame "TIC (OeLab)" {
            n185 = call "TIC_rw.vi"("write buffer"="in1.value?", "TIC 500"=w352) -> ("read buffer"=w355:string)  [unwired: 1 in, 2 out]
            n186 = Scan Value(string=w355, format string="%.3f") -> (value=w353:dbl)  [unwired: 1 in, 1 out]
          }
          frame "ITC" {
            n187 = local read "ITC signal"() -> (w358:T2)
            n188 = call "ITCGetReading.vi"("Signal"=w358) -> ("Reading"=w357:dbl)  [unwired: 6 in]
          }
          frame "ITC (SCPI)" {
            n189 = call "Isobus -BusCommandTimeout.vi"("Timeout (ms)"=u32 100, "Command"="READ:DEV:MB1.T1:TEMP:SIG:TEMP", "Address"=T7 {"Com Port"=1, "ISOBUS Address"=1, "GPIB Address"=25, "Communication"=enum."ISOBUS"}) -> ("Reply"=w364:string)  [unwired: 5 out]
            n190 = Match Pattern(string=w364, regular expression="SIG:TEMP:") -> (after substring=w362:string)  [unwired: 1 in, 3 out]
            n191 = Match Pattern(string=w362, regular expression="K") -> (before substring=w360:string)  [unwired: 1 in, 3 out]
            n192 = Fract/Exp String To Number(string=w360) -> (number=w359:dbl)  [unwired: 3 in, 1 out]
          }
          frame "GlobalVar" {
            n193 = global read "Tglobalvar.vi" "Tglobalvar"() -> (w368:dbl)
          }
        }
        "T [K]" <- w338
        n194 = Divide(x=w330, y=u32 100) -> (x/y=w328:dbl)
        "Time [s]" <- w328
        n195 = local read "Time"() -> (w332:dbl[])
        n196 = Build Array (concatenate)(w332, w328) -> (w333:dbl[])
        n197 = local write "Time"(w333) -> ()
        n198 = local read "B"() -> (w337:dbl[])
        n199 = Build Array (concatenate)(w337, w335) -> (w336:dbl[])
        n200 = local write "B"(w336) -> ()
        n201 = local read "T"() -> (w339:dbl[])
        n202 = Build Array (concatenate)(w339, w338) -> (w340:dbl[])
        n203 = local write "T"(w340) -> ()
      }
      frame "writeFile" {
        n204 = local read "SaveDataQuery"() -> (w369:bool)
        n205 = case shown="True" w369 {
          frame False {
          }
          frame True {
            w380 = "\t"
            w373 = "\t"
            w419 = "\t"
            w426 = "\t"
            w407 = "\t"
            w441 = "\t"
            w394 = "\t"
            w375 = "\r\n"
            w433 = "\t"
            # "Time\nT\nB\nWavelength\nDAC1\nDAC2\nDAC3\nDAC4\nV K2400_01\nV K2400_02\nLockin V\nLockin X\nLockin Y\nDMMX\nI K2400_01\nI K2400_02\n\nTime\nT\nB\nWavelength\nVsd\nVbgate\nVtopgate\nI2probe\nIleak bg\nIleak tg\nVxx\nVxy\nR2probe\nR4probe"
            # "I K2400_01\nI K2400_02"
            # "LK 1 X\nLK 1 Y\nLK2 X\nLK2 Y"
            # "DACs\nV K2400_01\nV K2400_02\nLockin V"
            # "Time\nT\nB\nWavelength"
            n206 = local read "DMM all (V)"() -> (w391:dbl[])
            n207 = local read "Wavelength [nm]"() -> (w435:dbl)
            n208 = local read "R 2probe [kOhm]"() -> (w414:dbl)
            n209 = local read "R 4probe [kOhm]"() -> (w413:dbl)
            n210 = local read "Lockin X all (V)"() -> (w382:dbl[])
            n211 = local read "V_backgate [V]"() -> (w430:dbl)
            n212 = local read "I Leak BG [nA]"() -> (w422:dbl)
            n213 = local read "V / I 3 [V or A]"() -> (w379:dbl)
            n214 = local read "V / I 4 [V or A]"() -> (w378:dbl)
            n215 = local read "V_topgate [V]"() -> (w429:dbl)
            n216 = local read "I Leak TG[nA]"() -> (w423:dbl)
            n217 = local read "I 2probe [nA]"() -> (w424:dbl)
            n218 = local read "T [K]"() -> (w449:dbl)
            n219 = local read "Time [s]"() -> (w451:dbl)
            n220 = local read "Vsd [V]"() -> (w432:dbl)
            n221 = local read "Vxy [V]"() -> (w415:dbl)
            n222 = local read "Vxx [V]"() -> (w416:dbl)
            n223 = Array Size(array=w391) -> (size(s)=w392:i32)
            n224 = local read "B [T]"() -> (w447:dbl)
            n225 = local read "Lockin A all (V)"() -> (w387:dbl[])
            n226 = local read "Lockin Y all (V)"() -> (w386:dbl[])
            n227 = for {
              N: w392 -> [_]
              tunnel: w391 -> [w468] mode=indexing
              tunnel: [w466] -> w390 mode=indexing
              n228 = Number To Exponential String(number=w468) -> (E-format string=w467:string)  [unwired: 3 in]
              n229 = Concatenate Strings(w467, "\t") -> (w466:string)
            }
            n230 = Array Size(array=w382) -> (size(s)=w381:i32)
            n231 = Number To Exponential String(number=w449) -> (E-format string=w448:string)  [unwired: 3 in]
            n232 = Number To Exponential String(number=w447) -> (E-format string=w446:string)  [unwired: 3 in]
            n233 = Number To Exponential String(number=w451) -> (E-format string=w450:string)  [unwired: 3 in]
            n234 = Number To Exponential String(number=w432) -> (E-format string=w431:string)  [unwired: 3 in]
            n235 = Number To Exponential String(number=w430) -> (E-format string=w428:string)  [unwired: 3 in]
            n236 = Number To Exponential String(number=w429) -> (E-format string=w427:string)  [unwired: 3 in]
            n237 = Number To Exponential String(number=w435) -> (E-format string=w434:string)  [unwired: 3 in]
            n238 = Number To Exponential String(number=w424) -> (E-format string=w418:string)  [unwired: 3 in]
            n239 = Number To Exponential String(number=w422) -> (E-format string=w420:string)  [unwired: 3 in]
            n240 = Number To Exponential String(number=w423) -> (E-format string=w421:string)  [unwired: 3 in]
            n241 = Number To Exponential String(number=w416) -> (E-format string=w412:string)  [unwired: 3 in]
            n242 = Number To Exponential String(number=w415) -> (E-format string=w411:string)  [unwired: 3 in]
            n243 = Number To Exponential String(number=w414) -> (E-format string=w410:string)  [unwired: 3 in]
            n244 = Number To Exponential String(number=w413) -> (E-format string=w409:string)  [unwired: 3 in]
            n245 = Number To Exponential String(number=w379) -> (E-format string=w377:string)  [unwired: 3 in]
            n246 = Number To Exponential String(number=w378) -> (E-format string=w376:string)  [unwired: 3 in]
            n247 = for {
              N: w381 -> [_]
              tunnel: w382 -> [w464] mode=indexing
              tunnel: [w462] -> w384 mode=indexing
              n248 = Number To Exponential String(number=w464) -> (E-format string=w463:string)  [unwired: 3 in]
              n249 = Concatenate Strings(w463, "\t") -> (w462:string)
            }
            n250 = for {
              N: w381 -> [_]
              tunnel: w386 -> [w456] mode=indexing
              tunnel: [w454] -> w383 mode=indexing
              n251 = Number To Exponential String(number=w456) -> (E-format string=w455:string)  [unwired: 3 in]
              n252 = Concatenate Strings(w455, "\t") -> (w454:string)
            }
            n253 = for {
              N: w381 -> [_]
              tunnel: w387 -> [w460] mode=indexing
              tunnel: [w458] -> w385 mode=indexing
              n254 = Number To Exponential String(number=w460) -> (E-format string=w459:string)  [unwired: 3 in]
              n255 = Concatenate Strings(w459, "\t") -> (w458:string)
            }
            n256 = Concatenate Strings(w431, w426, w428, w426, w427, w426) -> (w425:string)
            n257 = Concatenate Strings(w418, w419, w420, w419, w421, w419) -> (w417:string)
            n258 = Concatenate Strings(w412, w373, w411, w373, w410, w373, w409, w373) -> (w408:string)
            n259 = Concatenate Strings(w450, w433, w448, w433, w446, w433, w434, w433) -> (w399:string)
            n260 = Concatenate Strings(w377, w380, w376, w380) -> (w374:string)
            n261 = local read "refnum data"() -> (w452:refnum<file>)
            n262 = Concatenate Strings(w399, w425, w417, w408, w374, w375) -> (w436:string)
            n263 = local read "DAC 1 V [V]"() -> (w406:dbl)
            n264 = local read "DAC 2 V [V]"() -> (w404:dbl)
            n265 = local read "DAC 3 V [V]"() -> (w398:dbl)
            n266 = local read "DAC 4 V [V]"() -> (w397:dbl)
            n267 = local read "K2400 2 [V]"() -> (w443:dbl)
            n268 = local read "K2400 1 [V]"() -> (w445:dbl)
            n269 = Write to Text File(file (use dialog)=w452, text=w436) -> (error out=w401:errorcluster)  [unwired: 1 in, 3 out]
            n270 = Number To Exponential String(number=w443) -> (E-format string=w442:string)  [unwired: 3 in]
            n271 = Number To Exponential String(number=w406) -> (E-format string=w405:string)  [unwired: 3 in]
            n272 = Number To Exponential String(number=w404) -> (E-format string=w403:string)  [unwired: 3 in]
            n273 = Number To Exponential String(number=w398) -> (E-format string=w396:string)  [unwired: 3 in]
            n274 = Number To Exponential String(number=w397) -> (E-format string=w395:string)  [unwired: 3 in]
            n275 = Number To Exponential String(number=w445) -> (E-format string=w444:string)  [unwired: 3 in]
            n276 = local read "I K2400_2 [A]"() -> (w439:dbl)
            n277 = local read "I K2400_1 [A]"() -> (w440:dbl)
            n278 = Concatenate Strings(w405, w394, w403, w394, w396, w394, w395, w394, w444, w394, w442, w394, w385, w394) -> (w393:string)
            n279 = Concatenate Strings(w384, w441, w383, w441) -> (w388:string)
            n280 = Number To Exponential String(number=w439) -> (E-format string=w437:string)  [unwired: 3 in]
            n281 = Number To Exponential String(number=w440) -> (E-format string=w438:string)  [unwired: 3 in]
            n282 = Concatenate Strings(w390, w438, w407, w437, w407) -> (w389:string)
            n283 = local read "refnum raw"() -> (w402:refnum<file>)
            n284 = Concatenate Strings(w399, w393, w388, w389, w375) -> (w400:string)
            n285 = Write to Text File(file (use dialog)=w402, text=w400, error in=w401) -> ()  [unwired: 4 out]
          }
        }
        n286 = local read "Refresh Rate [ms]"() -> (w371:i32)
        n287 = call "wait.vi"("wait time (ms)"=w371) -> ("error in (no error) 2"=w370:errorcluster)  [unwired: 1 in]
      }
      frame "Calculate" {
        w505 = string[] ["Temperature", "B", "Wavelength", "Vsd", "Isd", "Vbg", "Vtg", "Ibg", "Itg", "Vxx", "Vxy", "R2probe", "R4probe", "Rxy", "VI3", "VI4"] ("Axis select")
        # "lockin1 X\nLockin2 X\nI K2400 01\nI K2400 02\nDMMxxx"
        # "DAC 1\nK2400 1\nK2400 2\nLockin\nDAC 2\nDAC 3\nDAC 4"
        n288 = local read "Gain Cluster 2"() -> (w544:T4)
        n289 = local read "signal cluster"() -> (w480:T1)
        n290 = local read "SetInstrument Cluster"() -> (w479:cluster{dbl, dbl, dbl, dbl[], dbl, dbl, dbl})
        n291 = Unbundle By Name(w544) -> ("Vsd"=w488:string, "I 2probe 2"=w486:string, "Vxx"=w491:string, "Vxy"=w489:string, "V BG"=w484:string, "I leak BG"=w496:string, "V TG"=w498:string, "I leak TG"=w494:string, "V / I 3"=w482:string, "V / I 4"=w481:string)
        n292 = Unbundle By Name(w544) -> ("I Gain 1"=w556:dbl, "V Gain 1"=w560:dbl, "conversion factor BG"=w558:dbl, "Vin / Vout 1"=w559:dbl, "V Gain 2"=w550:dbl, "Vin / Vout 2"=w549:dbl, "V Gain 3"=w548:dbl, "Vin / Vout 3"=w547:dbl, "I Gain 2"=w552:dbl, "I Gain 3"=w555:dbl, "conversion factor TG"=w546:dbl, "Vin / Vout 4"=w557:dbl, "Vin / Vout 5"=w545:dbl, "Manual Gain 1"=w551:dbl, "Manual Gain 2"=w553:dbl, "Manual Gain 3"=w554:dbl, "Gain V/I3"=w476:dbl, "Gain V/I4"=w475:dbl)
        n293 = call "SignalOutputV3.vi"("signal cluster 2"=w480, "Gain Type"=w484, "SetInstrument Cluster"=w479) -> ("Signal output"=w483:dbl)
        n294 = call "SignalOutputV3.vi"("signal cluster 2"=w480, "Gain Type"=w496, "SetInstrument Cluster"=w479) -> ("Signal output"=w495:dbl)
        n295 = call "SignalOutputV3.vi"("signal cluster 2"=w480, "Gain Type"=w498, "SetInstrument Cluster"=w479) -> ("Signal output"=w497:dbl)
        n296 = call "SignalOutputV3.vi"("signal cluster 2"=w480, "Gain Type"=w488, "SetInstrument Cluster"=w479) -> ("Signal output"=w487:dbl)
        n297 = call "SignalOutputV3.vi"("signal cluster 2"=w480, "Gain Type"=w486, "SetInstrument Cluster"=w479) -> ("Signal output"=w485:dbl)
        n298 = call "SignalOutputV3.vi"("signal cluster 2"=w480, "Gain Type"=w491, "SetInstrument Cluster"=w479) -> ("Signal output"=w492:dbl)
        n299 = call "SignalOutputV3.vi"("signal cluster 2"=w480, "Gain Type"=w489, "SetInstrument Cluster"=w479) -> ("Signal output"=w490:dbl)
        n300 = call "SignalOutputV3.vi"("signal cluster 2"=w480, "Gain Type"=w494, "SetInstrument Cluster"=w479) -> ("Signal output"=w493:dbl)
        n301 = call "SignalOutputV3.vi"("signal cluster 2"=w480, "Gain Type"=w482, "SetInstrument Cluster"=w479) -> ("Signal output"=w478:dbl)
        n302 = call "SignalOutputV3.vi"("signal cluster 2"=w480, "Gain Type"=w481, "SetInstrument Cluster"=w479) -> ("Signal output"=w477:dbl)
        n303 = Multiply(x=w560, y=w487) -> (x*y=w586:dbl)
        n304 = Multiply(x=w483, y=w558) -> (x*y=w579:dbl)
        n305 = Divide(x=w485, y=w556) -> (x/y=w584:dbl)
        n306 = Divide(x=w492, y=w550) -> (x/y=w581:dbl)
        n307 = Divide(x=w490, y=w548) -> (x/y=w580:dbl)
        n308 = Divide(x=w495, y=w552) -> (x/y=w583:dbl)
        n309 = Multiply(x=w497, y=w546) -> (x*y=w578:dbl)
        n310 = Divide(x=w493, y=w555) -> (x/y=w582:dbl)
        n311 = Multiply(x=w478, y=w476) -> (x*y=w474:dbl)
        "V / I 3 [V or A]" <- w474
        n312 = Multiply(x=w477, y=w475) -> (x*y=w473:dbl)
        "V / I 4 [V or A]" <- w473
        n313 = Multiply(x=w583, y=w553) -> (x*y=w563:dbl)
        n314 = Multiply(x=w582, y=w554) -> (x*y=w575:dbl)
        n315 = Multiply(x=w586, y=w559) -> (x*y=w577:dbl)
        "Vsd [V]" <- w577
        n316 = Multiply(x=w581, y=w549) -> (x*y=w571:dbl)
        "Vxx [V]" <- w571
        n317 = Multiply(x=w580, y=w547) -> (x*y=w536:dbl)
        "Vxy [V]" <- w536
        n318 = Multiply(x=w579, y=w557) -> (x*y=w569:dbl)
        "V_backgate [V]" <- w569
        n319 = Multiply(x=w578, y=w545) -> (x*y=w567:dbl)
        "V_topgate [V]" <- w567
        n320 = Multiply(x=w584, y=w551) -> (x*y=w534:dbl)
        n321 = Multiply(x=w563, y=1000000000.0) -> (x*y=w562:dbl)
        "I Leak BG [nA]" <- w562
        n322 = Multiply(x=w575, y=1000000000.0) -> (x*y=w566:dbl)
        "I Leak TG[nA]" <- w566
        n323 = Multiply(x=w534, y=1000000000.0) -> (x*y=w535:dbl)
        "I 2probe [nA]" <- w535
        n324 = Divide(x=w577, y=w535) -> (x/y=w543:dbl)
        n325 = Divide(x=w536, y=w534) -> (x/y=w533:dbl)
        n326 = Divide(x=w571, y=w535) -> (x/y=w539:dbl)
        n327 = Divide(x=w533, y=1000.0) -> (x/y=w531:dbl)
        n328 = local read "R2probe array"() -> (w573:dbl[])
        n329 = local read "R4probe array"() -> (w572:dbl[])
        n330 = local read "Rxy Array"() -> (w537:dbl[])
        n331 = local read "Vbg array"() -> (w525:dbl[])
        n332 = local read "V/I3 array"() -> (w471:dbl[])
        n333 = local read "V/I4 array"() -> (w472:dbl[])
        n334 = local read "Vsd array"() -> (w527:dbl[])
        n335 = local read "Vxy array"() -> (w568:dbl[])
        n336 = local read "Vtg array"() -> (w524:dbl[])
        n337 = local read "Ibg array"() -> (w574:dbl[])
        n338 = local read "Vxx array"() -> (w570:dbl[])
        n339 = local read "Isd array"() -> (w526:dbl[])
        n340 = local read "Itg array"() -> (w576:dbl[])
        n341 = Multiply(x=w543, y=1000000.0) -> (x*y=w541:dbl)
        "R 2probe [kOhm]" <- w541
        n342 = Multiply(x=w539, y=1000000.0) -> (x*y=w538:dbl)
        "R 4probe [kOhm]" <- w538
        n343 = local read "Wavelength array"() -> (w528:dbl[])
        n344 = Build Array (concatenate)(w527, w577) -> (w523:dbl[])
        n345 = Build Array (concatenate)(w568, w536) -> (w516:dbl[])
        n346 = Build Array (concatenate)(w573, w541) -> (w515:dbl[])
        n347 = Build Array (concatenate)(w537, w531) -> (w513:dbl[])
        n348 = Build Array (concatenate)(w570, w571) -> (w517:dbl[])
        n349 = Build Array (concatenate)(w525, w569) -> (w521:dbl[])
        n350 = Build Array (concatenate)(w524, w567) -> (w520:dbl[])
        n351 = Build Array (concatenate)(w526, w535) -> (w522:dbl[])
        n352 = Build Array (concatenate)(w572, w538) -> (w514:dbl[])
        n353 = Build Array (concatenate)(w574, w562) -> (w519:dbl[])
        n354 = Build Array (concatenate)(w576, w566) -> (w518:dbl[])
        n355 = Build Array (concatenate)(w471, w474) -> (w470:dbl[])
        n356 = Build Array (concatenate)(w472, w473) -> (w469:dbl[])
        n357 = local write "Vsd array"(w523) -> ()
        n358 = local write "Vxy array"(w516) -> ()
        n359 = local write "R2probe array"(w515) -> ()
        n360 = local write "Rxy Array"(w513) -> ()
        n361 = local write "Vxx array"(w517) -> ()
        n362 = local write "Vbg array"(w521) -> ()
        n363 = local write "Vtg array"(w520) -> ()
        n364 = local write "Isd array"(w522) -> ()
        n365 = local write "R4probe array"(w514) -> ()
        n366 = local write "Ibg array"(w519) -> ()
        n367 = local write "Itg array"(w518) -> ()
        n368 = local write "V/I3 array"(w470) -> ()
        n369 = local read "T"() -> (w530:dbl[])
        n370 = local read "B"() -> (w529:dbl[])
        n371 = local write "V/I4 array"(w469) -> ()
        n372 = Build Array(w530, w529, w528, w523, w522, w521, w520, w519, w518, w517, w516, w515, w514, w513, w470, w469) -> (w506:dbl[][])
        n373 = call "Evalmutlivar.vi"("Variables"=w505, "Matrix data"=w506, "formula"="Formula 4") -> ("error out"=w499:errorcluster, "Y Values"=→"Formula4Array":dbl[])  [unwired: 1 in]
        n374 = call "Evalmutlivar.vi"("Variables"=w505, "Matrix data"=w506, "formula"="Formula 1") -> ("error out"=w511:errorcluster, "Y Values"=→"Formula1Array":dbl[])  [unwired: 1 in]
        n375 = call "Evalmutlivar.vi"("Variables"=w505, "Matrix data"=w506, "formula"="Formula 2") -> ("error out"=w501:errorcluster, "Y Values"=→"Formula2Array":dbl[])  [unwired: 1 in]
        n376 = call "Evalmutlivar.vi"("Variables"=w505, "Matrix data"=w506, "formula"="Formula 3") -> ("error out"=w500:errorcluster, "Y Values"=→"Formula3Array":dbl[])  [unwired: 1 in]
      }
      frame "stop" {
        n377 = local read "refnum data"() -> (w588:refnum<file>)
        n378 = local read "refnum raw"() -> (w587:refnum<file>)
        n379 = Close File(refnum=w588) -> ()  [unwired: 1 in, 2 out]
        n380 = Close File(refnum=w587) -> ()  [unwired: 1 in, 2 out]
      }
    }
    n381 = global read "stopButton.vi" "stopsignal"() -> (w35:bool)
    n382 = local write "stop"(w35) -> ()
    n383 = Unbundle By Name("Device Cluster") -> ("K2400 1"=→"K2400 1":refnum<visa-resource-name>, "K2400_1"=→"K2400_1":bool, "K2400 2"=→"K2400 2":refnum<visa-resource-name>, "K2400_2"=→"K2400_2":bool, "LockinX"=→"LockinX":string[][], "TIC"=→"TIC":refnum<visa-resource-name>, "Tcontrol"=→"Tcontrol":string, "DMMX"=→"DMMX":string[][], "DAC"=→"DAC":refnum<visa-resource-name>, "DAC present"=→"DAC present":bool, "Bfield query"=→"Bfield query":bool, "Wvlen query"=→"Wvlen query":bool, "ITC signal"=→"ITC signal":T2)
    n384 = Or(x=w38, y="stop") -> (x .or. y?=w36:bool)
    "stopMainLoop" <- w36
  }
  n385 = Array Size(array=w14) -> (size(s)=w15:i32[])
  n386 = Array Size(array=w4) -> (size(s)=w8:i32[])
  n387 = Index Array(array=w15, index=0) -> (element=w13:i32)
  n388 = Index Array(array=w8, index=0) -> (element=w3:i32)
  n389 = for {
    N: w13 -> [_]
    tunnel: w14 -> [_] mode=indexing
    tunnel: [w591] -> w11 mode=indexing
    i -> [w594]
    n390 = Increment(x=w594) -> (x+1=w592:i32)
    n391 = Number To Decimal String(number=w592) -> (decimal integer string=w593:string)  [unwired: 1 in]
    n392 = Concatenate Strings("DMM", w593) -> (w591:string)
  }
  n393 = for {
    N: w3 -> [_]
    tunnel: w4 -> [_] mode=indexing
    tunnel: [w596] -> w6 mode=indexing
    i -> [w599]
    n394 = Increment(x=w599) -> (x+1=w597:i32)
    n395 = Number To Decimal String(number=w597) -> (decimal integer string=w598:string)  [unwired: 1 in]
    n396 = Concatenate Strings("X Lockin", w598) -> (w596:string)
  }
  n397 = for {
    N: w3 -> [_]
    tunnel: [w601] -> w5 mode=indexing
    tunnel: w4 -> [_] mode=indexing
    i -> [w604]
    n398 = Increment(x=w604) -> (x+1=w602:i32)
    n399 = Number To Decimal String(number=w602) -> (decimal integer string=w603:string)  [unwired: 1 in]
    n400 = Concatenate Strings("Y Lockin", w603) -> (w601:string)
  }
  n401 = for {
    N: w3 -> [_]
    tunnel: [w606] -> w2 mode=indexing
    tunnel: w4 -> [_] mode=indexing
    i -> [w609]
    n402 = Increment(x=w609) -> (x+1=w607:i32)
    n403 = Number To Decimal String(number=w607) -> (decimal integer string=w608:string)  [unwired: 1 in]
    n404 = Concatenate Strings("Am Lockin", w608) -> (w606:string)
  }
  n405 = while {
    shift-right: [w651] -> _
    shift-left: "plot" -> [w652]
    tunnel: w10 -> [w628]
    tunnel: w9 -> [w627]
    stop <- w653 stop-if-true
    n406 = local read "Refresh Rate [ms]"() -> (w631:i32)
    n407 = case shown="\"Itg\"" "X-Axis 3" {
      selector: "X-Axis 3" -> [_ _ _ _ _ _ _ _ _ _ _ _ _ _ _ _ _ _ _ _ _ _ _ w746 w754 w762 w770 _ _ _ _ _ _]
      tunnel: [w716 w717 w718 w719 w720 w721 w722 w723 w724 w725 w726 w727 w728 w729 w730 w731 w732 w733 w734 w735 w736 w737 w738 w740 w748 w756 w764 w771 w772 w773 w774 w775 w776] -> w614
      frame "DAC 1 V", Default {
        n408 = local read "DAC 1 array"() -> (w716:dbl[])
      }
      frame "DAC 2 V" {
        n409 = local read "DAC 2 array"() -> (w717:dbl[])
      }
      frame "DAC 3 V" {
        n410 = local read "DAC 3 array"() -> (w718:dbl[])
      }
      frame "DAC 4 V" {
        n411 = local read "DAC 4 array"() -> (w719:dbl[])
      }
      frame "Wavelength" {
        n412 = local read "Wavelength array"() -> (w720:dbl[])
      }
      frame "Vsd" {
        n413 = local read "Vsd array"() -> (w721:dbl[])
      }
      frame "Isd" {
        n414 = local read "Isd array"() -> (w722:dbl[])
      }
      frame "Vbg" {
        n415 = local read "Vbg array"() -> (w723:dbl[])
      }
      frame "Vtg" {
        n416 = local read "Vtg array"() -> (w724:dbl[])
      }
      frame "Ibg" {
        n417 = local read "Ibg array"() -> (w725:dbl[])
      }
      frame "Itg" {
        n418 = local read "Itg array"() -> (w726:dbl[])
      }
      frame "Vxx" {
        n419 = local read "Vxx array"() -> (w727:dbl[])
      }
      frame "Vxy" {
        n420 = local read "Vxy array"() -> (w728:dbl[])
      }
      frame "V/I 3" {
        n421 = local read "V/I3 array"() -> (w729:dbl[])
      }
      frame "V/I 4" {
        n422 = local read "V/I4 array"() -> (w730:dbl[])
      }
      frame "Rxy" {
        n423 = local read "Rxy Array"() -> (w731:dbl[])
      }
      frame "R2probe" {
        n424 = local read "R2probe array"() -> (w732:dbl[])
      }
      frame "Temperature" {
        n425 = local read "T"() -> (w733:dbl[])
      }
      frame "time" {
        n426 = local read "Time"() -> (w734:dbl[])
      }
      frame "V K2400_01" {
        n427 = local read "V K2400_01 array"() -> (w735:dbl[])
      }
      frame "V K2400_02" {
        n428 = local read "V K2400_02 array"() -> (w736:dbl[])
      }
      frame "I K2400_01" {
        n429 = local read "I K2400 01"() -> (w737:dbl[])
      }
      frame "I K2400_02" {
        n430 = local read "I K2400 02"() -> (w738:dbl[])
      }
      frame "DMM1".."DMM9" {
        n431 = Match Pattern(string=w746, regular expression="DMM") -> (after substring=w744:string)  [unwired: 1 in, 3 out]
        n432 = Scan Value(string=w744, format string="%g") -> (value=w741:dbl)  [unwired: 1 in, 1 out]
        n433 = local read "DMM Array"() -> (w742:dbl[][])
        n434 = Decrement(x=w741) -> (x-1=w739:dbl)
        n435 = Index Array(array=w742, index (col)=w739) -> (element=w740:dbl[])  [unwired: 1 in]
      }
      frame "X Lockin1".."X Lockin9" {
        n436 = Match Pattern(string=w754, regular expression="X Lockin") -> (after substring=w752:string)  [unwired: 1 in, 3 out]
        n437 = local read "Lockin X Array"() -> (w750:dbl[][])
        n438 = Scan Value(string=w752, format string="%g") -> (value=w749:dbl)  [unwired: 1 in, 1 out]
        n439 = Decrement(x=w749) -> (x-1=w747:dbl)
        n440 = Index Array(array=w750, index (col)=w747) -> (element=w748:dbl[])  [unwired: 1 in]
      }
      frame "Y Lockin1".."Y Lockin9" {
        n441 = Match Pattern(string=w762, regular expression="Y Lockin") -> (after substring=w760:string)  [unwired: 1 in, 3 out]
        n442 = local read "Lockin Y Array"() -> (w758:dbl[][])
        n443 = Scan Value(string=w760, format string="%g") -> (value=w757:dbl)  [unwired: 1 in, 1 out]
        n444 = Decrement(x=w757) -> (x-1=w755:dbl)
        n445 = Index Array(array=w758, index (col)=w755) -> (element=w756:dbl[])  [unwired: 1 in]
      }
      frame "Am Lockin1".."Am Lockin9" {
        n446 = local read "Lockin A Array"() -> (w766:dbl[][])
        n447 = Match Pattern(string=w770, regular expression="Am Lockin") -> (after substring=w768:string)  [unwired: 1 in, 3 out]
        n448 = Scan Value(string=w768, format string="%g") -> (value=w765:dbl)  [unwired: 1 in, 1 out]
        n449 = Decrement(x=w765) -> (x-1=w763:dbl)
        n450 = Index Array(array=w766, index (col)=w763) -> (element=w764:dbl[])  [unwired: 1 in]
      }
      frame "B" {
        n451 = local read "B"() -> (w771:dbl[])
      }
      frame "R4probe" {
        n452 = local read "R4probe array"() -> (w772:dbl[])
      }
      frame "Formula1" {
        n453 = local read "Formula1Array"() -> (w773:dbl[])
      }
      frame "Formula2" {
        n454 = local read "Formula2Array"() -> (w774:dbl[])
      }
      frame "Formula3" {
        n455 = local read "Formula3Array"() -> (w775:dbl[])
      }
      frame "Formula4" {
        n456 = local read "Formula4Array"() -> (w776:dbl[])
      }
    }
    n457 = case shown="\"Itg\"" "Y-Axis 3" {
      selector: "Y-Axis 3" -> [_ _ _ _ _ _ _ _ _ _ _ _ _ _ _ _ _ _ _ _ _ _ _ w685 w693 w701 w709 _ _ _ _ _ _]
      tunnel: [w655 w656 w657 w658 w659 w660 w661 w662 w663 w664 w665 w666 w667 w668 w669 w670 w671 w672 w673 w674 w675 w676 w677 w679 w687 w695 w703 w710 w711 w712 w713 w714 w715] -> w611
      frame "DAC 1 V", Default {
        n458 = local read "DAC 1 array"() -> (w655:dbl[])
      }
      frame "DAC 2 V" {
        n459 = local read "DAC 2 array"() -> (w656:dbl[])
      }
      frame "DAC 3 V" {
        n460 = local read "DAC 3 array"() -> (w657:dbl[])
      }
      frame "DAC 4 V" {
        n461 = local read "DAC 4 array"() -> (w658:dbl[])
      }
      frame "Wavelength" {
        n462 = local read "Wavelength array"() -> (w659:dbl[])
      }
      frame "Vsd" {
        n463 = local read "Vsd array"() -> (w660:dbl[])
      }
      frame "Isd" {
        n464 = local read "Isd array"() -> (w661:dbl[])
      }
      frame "Vbg" {
        n465 = local read "Vbg array"() -> (w662:dbl[])
      }
      frame "Vtg" {
        n466 = local read "Vtg array"() -> (w663:dbl[])
      }
      frame "Ibg" {
        n467 = local read "Ibg array"() -> (w664:dbl[])
      }
      frame "Itg" {
        n468 = local read "Itg array"() -> (w665:dbl[])
      }
      frame "Vxx" {
        n469 = local read "Vxx array"() -> (w666:dbl[])
      }
      frame "Vxy" {
        n470 = local read "Vxy array"() -> (w667:dbl[])
      }
      frame "V/I 3" {
        n471 = local read "V/I3 array"() -> (w668:dbl[])
      }
      frame "V/I 4" {
        n472 = local read "V/I4 array"() -> (w669:dbl[])
      }
      frame "Rxy" {
        n473 = local read "Rxy Array"() -> (w670:dbl[])
      }
      frame "R2probe" {
        n474 = local read "R2probe array"() -> (w671:dbl[])
      }
      frame "Temperature" {
        n475 = local read "T"() -> (w672:dbl[])
      }
      frame "time" {
        n476 = local read "Time"() -> (w673:dbl[])
      }
      frame "V K2400_01" {
        n477 = local read "V K2400_01 array"() -> (w674:dbl[])
      }
      frame "V K2400_02" {
        n478 = local read "V K2400_02 array"() -> (w675:dbl[])
      }
      frame "I K2400_01" {
        n479 = local read "I K2400 01"() -> (w676:dbl[])
      }
      frame "I K2400_02" {
        n480 = local read "I K2400 02"() -> (w677:dbl[])
      }
      frame "DMM1".."DMM9" {
        n481 = Match Pattern(string=w685, regular expression="DMM") -> (after substring=w683:string)  [unwired: 1 in, 3 out]
        n482 = Scan Value(string=w683, format string="%g") -> (value=w680:dbl)  [unwired: 1 in, 1 out]
        n483 = local read "DMM Array"() -> (w681:dbl[][])
        n484 = Decrement(x=w680) -> (x-1=w678:dbl)
        n485 = Index Array(array=w681, index (col)=w678) -> (element=w679:dbl[])  [unwired: 1 in]
      }
      frame "X Lockin1".."X Lockin9" {
        n486 = Match Pattern(string=w693, regular expression="X Lockin") -> (after substring=w691:string)  [unwired: 1 in, 3 out]
        n487 = local read "Lockin X Array"() -> (w689:dbl[][])
        n488 = Scan Value(string=w691, format string="%g") -> (value=w688:dbl)  [unwired: 1 in, 1 out]
        n489 = Decrement(x=w688) -> (x-1=w686:dbl)
        n490 = Index Array(array=w689, index (col)=w686) -> (element=w687:dbl[])  [unwired: 1 in]
      }
      frame "Y Lockin1".."Y Lockin9" {
        n491 = Match Pattern(string=w701, regular expression="Y Lockin") -> (after substring=w699:string)  [unwired: 1 in, 3 out]
        n492 = local read "Lockin Y Array"() -> (w697:dbl[][])
        n493 = Scan Value(string=w699, format string="%g") -> (value=w696:dbl)  [unwired: 1 in, 1 out]
        n494 = Decrement(x=w696) -> (x-1=w694:dbl)
        n495 = Index Array(array=w697, index (col)=w694) -> (element=w695:dbl[])  [unwired: 1 in]
      }
      frame "Am Lockin1".."Am Lockin9" {
        n496 = local read "Lockin A Array"() -> (w705:dbl[][])
        n497 = Match Pattern(string=w709, regular expression="Am Lockin") -> (after substring=w707:string)  [unwired: 1 in, 3 out]
        n498 = Scan Value(string=w707, format string="%g") -> (value=w704:dbl)  [unwired: 1 in, 1 out]
        n499 = Decrement(x=w704) -> (x-1=w702:dbl)
        n500 = Index Array(array=w705, index (col)=w702) -> (element=w703:dbl[])  [unwired: 1 in]
      }
      frame "B" {
        n501 = local read "B"() -> (w710:dbl[])
      }
      frame "R4probe" {
        n502 = local read "R4probe array"() -> (w711:dbl[])
      }
      frame "Formula1" {
        n503 = local read "Formula1Array"() -> (w712:dbl[])
      }
      frame "Formula2" {
        n504 = local read "Formula2Array"() -> (w713:dbl[])
      }
      frame "Formula3" {
        n505 = local read "Formula3Array"() -> (w714:dbl[])
      }
      frame "Formula4" {
        n506 = local read "Formula4Array"() -> (w715:dbl[])
      }
    }
    n507 = call "AxisLabel.vi"("Axis"="X-Axis 3") -> ("X Scale.Name Label.Text"=w639:string)
    n508 = call "AxisLabel.vi"("Axis"="Y-Axis 3") -> ("X Scale.Name Label.Text"=w638:string)
    n509 = case shown="\"Itg\"" "X-Axis 4" {
      selector: "X-Axis 4" -> [_ _ _ _ _ _ _ _ _ _ _ _ _ _ _ _ _ _ _ _ _ _ _ w1112 w1120 w1128 w1136 _ _ _ _ _ _]
      tunnel: [w1082 w1083 w1084 w1085 w1086 w1087 w1088 w1089 w1090 w1091 w1092 w1093 w1094 w1095 w1096 w1097 w1098 w1099 w1100 w1101 w1102 w1103 w1104 w1106 w1114 w1122 w1130 w1137 w1138 w1139 w1140 w1141 w1142] -> w625
      frame "DAC 1 V", Default {
        n510 = local read "DAC 1 array"() -> (w1082:dbl[])
      }
      frame "DAC 2 V" {
        n511 = local read "DAC 2 array"() -> (w1083:dbl[])
      }
      frame "DAC 3 V" {
        n512 = local read "DAC 3 array"() -> (w1084:dbl[])
      }
      frame "DAC 4 V" {
        n513 = local read "DAC 4 array"() -> (w1085:dbl[])
      }
      frame "Wavelength" {
        n514 = local read "Wavelength array"() -> (w1086:dbl[])
      }
      frame "Vsd" {
        n515 = local read "Vsd array"() -> (w1087:dbl[])
      }
      frame "Isd" {
        n516 = local read "Isd array"() -> (w1088:dbl[])
      }
      frame "Vbg" {
        n517 = local read "Vbg array"() -> (w1089:dbl[])
      }
      frame "Vtg" {
        n518 = local read "Vtg array"() -> (w1090:dbl[])
      }
      frame "Ibg" {
        n519 = local read "Ibg array"() -> (w1091:dbl[])
      }
      frame "Itg" {
        n520 = local read "Itg array"() -> (w1092:dbl[])
      }
      frame "Vxx" {
        n521 = local read "Vxx array"() -> (w1093:dbl[])
      }
      frame "Vxy" {
        n522 = local read "Vxy array"() -> (w1094:dbl[])
      }
      frame "V/I 3" {
        n523 = local read "V/I3 array"() -> (w1095:dbl[])
      }
      frame "V/I 4" {
        n524 = local read "V/I4 array"() -> (w1096:dbl[])
      }
      frame "Rxy" {
        n525 = local read "Rxy Array"() -> (w1097:dbl[])
      }
      frame "R2probe" {
        n526 = local read "R2probe array"() -> (w1098:dbl[])
      }
      frame "Temperature" {
        n527 = local read "T"() -> (w1099:dbl[])
      }
      frame "time" {
        n528 = local read "Time"() -> (w1100:dbl[])
      }
      frame "V K2400_01" {
        n529 = local read "V K2400_01 array"() -> (w1101:dbl[])
      }
      frame "V K2400_02" {
        n530 = local read "V K2400_02 array"() -> (w1102:dbl[])
      }
      frame "I K2400_01" {
        n531 = local read "I K2400 01"() -> (w1103:dbl[])
      }
      frame "I K2400_02" {
        n532 = local read "I K2400 02"() -> (w1104:dbl[])
      }
      frame "DMM1".."DMM9" {
        n533 = Match Pattern(string=w1112, regular expression="DMM") -> (after substring=w1110:string)  [unwired: 1 in, 3 out]
        n534 = Scan Value(string=w1110, format string="%g") -> (value=w1107:dbl)  [unwired: 1 in, 1 out]
        n535 = local read "DMM Array"() -> (w1108:dbl[][])
        n536 = Decrement(x=w1107) -> (x-1=w1105:dbl)
        n537 = Index Array(array=w1108, index (col)=w1105) -> (element=w1106:dbl[])  [unwired: 1 in]
      }
      frame "X Lockin1".."X Lockin9" {
        n538 = Match Pattern(string=w1120, regular expression="X Lockin") -> (after substring=w1118:string)  [unwired: 1 in, 3 out]
        n539 = local read "Lockin X Array"() -> (w1116:dbl[][])
        n540 = Scan Value(string=w1118, format string="%g") -> (value=w1115:dbl)  [unwired: 1 in, 1 out]
        n541 = Decrement(x=w1115) -> (x-1=w1113:dbl)
        n542 = Index Array(array=w1116, index (col)=w1113) -> (element=w1114:dbl[])  [unwired: 1 in]
      }
      frame "Y Lockin1".."Y Lockin9" {
        n543 = Match Pattern(string=w1128, regular expression="Y Lockin") -> (after substring=w1126:string)  [unwired: 1 in, 3 out]
        n544 = local read "Lockin Y Array"() -> (w1124:dbl[][])
        n545 = Scan Value(string=w1126, format string="%g") -> (value=w1123:dbl)  [unwired: 1 in, 1 out]
        n546 = Decrement(x=w1123) -> (x-1=w1121:dbl)
        n547 = Index Array(array=w1124, index (col)=w1121) -> (element=w1122:dbl[])  [unwired: 1 in]
      }
      frame "Am Lockin1".."Am Lockin9" {
        n548 = local read "Lockin A Array"() -> (w1132:dbl[][])
        n549 = Match Pattern(string=w1136, regular expression="Am Lockin") -> (after substring=w1134:string)  [unwired: 1 in, 3 out]
        n550 = Scan Value(string=w1134, format string="%g") -> (value=w1131:dbl)  [unwired: 1 in, 1 out]
        n551 = Decrement(x=w1131) -> (x-1=w1129:dbl)
        n552 = Index Array(array=w1132, index (col)=w1129) -> (element=w1130:dbl[])  [unwired: 1 in]
      }
      frame "B" {
        n553 = local read "B"() -> (w1137:dbl[])
      }
      frame "R4probe" {
        n554 = local read "R4probe array"() -> (w1138:dbl[])
      }
      frame "Formula1" {
        n555 = local read "Formula1Array"() -> (w1139:dbl[])
      }
      frame "Formula2" {
        n556 = local read "Formula2Array"() -> (w1140:dbl[])
      }
      frame "Formula3" {
        n557 = local read "Formula3Array"() -> (w1141:dbl[])
      }
      frame "Formula4" {
        n558 = local read "Formula4Array"() -> (w1142:dbl[])
      }
    }
    n559 = case shown="\"Itg\"" "Y-Axis 4" {
      selector: "Y-Axis 4" -> [_ _ _ _ _ _ _ _ _ _ _ _ _ _ _ _ _ _ _ _ _ _ _ w1051 w1059 w1067 w1075 _ _ _ _ _ _]
      tunnel: [w1021 w1022 w1023 w1024 w1025 w1026 w1027 w1028 w1029 w1030 w1031 w1032 w1033 w1034 w1035 w1036 w1037 w1038 w1039 w1040 w1041 w1042 w1043 w1045 w1053 w1061 w1069 w1076 w1077 w1078 w1079 w1080 w1081] -> w623
      frame "DAC 1 V", Default {
        n560 = local read "DAC 1 array"() -> (w1021:dbl[])
      }
      frame "DAC 2 V" {
        n561 = local read "DAC 2 array"() -> (w1022:dbl[])
      }
      frame "DAC 3 V" {
        n562 = local read "DAC 3 array"() -> (w1023:dbl[])
      }
      frame "DAC 4 V" {
        n563 = local read "DAC 4 array"() -> (w1024:dbl[])
      }
      frame "Wavelength" {
        n564 = local read "Wavelength array"() -> (w1025:dbl[])
      }
      frame "Vsd" {
        n565 = local read "Vsd array"() -> (w1026:dbl[])
      }
      frame "Isd" {
        n566 = local read "Isd array"() -> (w1027:dbl[])
      }
      frame "Vbg" {
        n567 = local read "Vbg array"() -> (w1028:dbl[])
      }
      frame "Vtg" {
        n568 = local read "Vtg array"() -> (w1029:dbl[])
      }
      frame "Ibg" {
        n569 = local read "Ibg array"() -> (w1030:dbl[])
      }
      frame "Itg" {
        n570 = local read "Itg array"() -> (w1031:dbl[])
      }
      frame "Vxx" {
        n571 = local read "Vxx array"() -> (w1032:dbl[])
      }
      frame "Vxy" {
        n572 = local read "Vxy array"() -> (w1033:dbl[])
      }
      frame "V/I 3" {
        n573 = local read "V/I3 array"() -> (w1034:dbl[])
      }
      frame "V/I 4" {
        n574 = local read "V/I4 array"() -> (w1035:dbl[])
      }
      frame "Rxy" {
        n575 = local read "Rxy Array"() -> (w1036:dbl[])
      }
      frame "R2probe" {
        n576 = local read "R2probe array"() -> (w1037:dbl[])
      }
      frame "Temperature" {
        n577 = local read "T"() -> (w1038:dbl[])
      }
      frame "time" {
        n578 = local read "Time"() -> (w1039:dbl[])
      }
      frame "V K2400_01" {
        n579 = local read "V K2400_01 array"() -> (w1040:dbl[])
      }
      frame "V K2400_02" {
        n580 = local read "V K2400_02 array"() -> (w1041:dbl[])
      }
      frame "I K2400_01" {
        n581 = local read "I K2400 01"() -> (w1042:dbl[])
      }
      frame "I K2400_02" {
        n582 = local read "I K2400 02"() -> (w1043:dbl[])
      }
      frame "DMM1".."DMM9" {
        n583 = Match Pattern(string=w1051, regular expression="DMM") -> (after substring=w1049:string)  [unwired: 1 in, 3 out]
        n584 = Scan Value(string=w1049, format string="%g") -> (value=w1046:dbl)  [unwired: 1 in, 1 out]
        n585 = local read "DMM Array"() -> (w1047:dbl[][])
        n586 = Decrement(x=w1046) -> (x-1=w1044:dbl)
        n587 = Index Array(array=w1047, index (col)=w1044) -> (element=w1045:dbl[])  [unwired: 1 in]
      }
      frame "X Lockin1".."X Lockin9" {
        n588 = Match Pattern(string=w1059, regular expression="X Lockin") -> (after substring=w1057:string)  [unwired: 1 in, 3 out]
        n589 = local read "Lockin X Array"() -> (w1055:dbl[][])
        n590 = Scan Value(string=w1057, format string="%g") -> (value=w1054:dbl)  [unwired: 1 in, 1 out]
        n591 = Decrement(x=w1054) -> (x-1=w1052:dbl)
        n592 = Index Array(array=w1055, index (col)=w1052) -> (element=w1053:dbl[])  [unwired: 1 in]
      }
      frame "Y Lockin1".."Y Lockin9" {
        n593 = Match Pattern(string=w1067, regular expression="Y Lockin") -> (after substring=w1065:string)  [unwired: 1 in, 3 out]
        n594 = local read "Lockin Y Array"() -> (w1063:dbl[][])
        n595 = Scan Value(string=w1065, format string="%g") -> (value=w1062:dbl)  [unwired: 1 in, 1 out]
        n596 = Decrement(x=w1062) -> (x-1=w1060:dbl)
        n597 = Index Array(array=w1063, index (col)=w1060) -> (element=w1061:dbl[])  [unwired: 1 in]
      }
      frame "Am Lockin1".."Am Lockin9" {
        n598 = local read "Lockin A Array"() -> (w1071:dbl[][])
        n599 = Match Pattern(string=w1075, regular expression="Am Lockin") -> (after substring=w1073:string)  [unwired: 1 in, 3 out]
        n600 = Scan Value(string=w1073, format string="%g") -> (value=w1070:dbl)  [unwired: 1 in, 1 out]
        n601 = Decrement(x=w1070) -> (x-1=w1068:dbl)
        n602 = Index Array(array=w1071, index (col)=w1068) -> (element=w1069:dbl[])  [unwired: 1 in]
      }
      frame "B" {
        n603 = local read "B"() -> (w1076:dbl[])
      }
      frame "R4probe" {
        n604 = local read "R4probe array"() -> (w1077:dbl[])
      }
      frame "Formula1" {
        n605 = local read "Formula1Array"() -> (w1078:dbl[])
      }
      frame "Formula2" {
        n606 = local read "Formula2Array"() -> (w1079:dbl[])
      }
      frame "Formula3" {
        n607 = local read "Formula3Array"() -> (w1080:dbl[])
      }
      frame "Formula4" {
        n608 = local read "Formula4Array"() -> (w1081:dbl[])
      }
    }
    n609 = call "AxisLabel.vi"("Axis"="X-Axis 2") -> ("X Scale.Name Label.Text"=w649:string)
    n610 = case shown="\"Itg\"" "X-Axis 2" {
      selector: "X-Axis 2" -> [_ _ _ _ _ _ _ _ _ _ _ _ _ _ _ _ _ _ _ _ _ _ _ w990 w998 w1006 w1014 _ _ _ _ _ _]
      tunnel: [w960 w961 w962 w963 w964 w965 w966 w967 w968 w969 w970 w971 w972 w973 w974 w975 w976 w977 w978 w979 w980 w981 w982 w984 w992 w1000 w1008 w1015 w1016 w1017 w1018 w1019 w1020] -> w622
      frame "DAC 1 V", Default {
        n611 = local read "DAC 1 array"() -> (w960:dbl[])
      }
      frame "DAC 2 V" {
        n612 = local read "DAC 2 array"() -> (w961:dbl[])
      }
      frame "DAC 3 V" {
        n613 = local read "DAC 3 array"() -> (w962:dbl[])
      }
      frame "DAC 4 V" {
        n614 = local read "DAC 4 array"() -> (w963:dbl[])
      }
      frame "Wavelength" {
        n615 = local read "Wavelength array"() -> (w964:dbl[])
      }
      frame "Vsd" {
        n616 = local read "Vsd array"() -> (w965:dbl[])
      }
      frame "Isd" {
        n617 = local read "Isd array"() -> (w966:dbl[])
      }
      frame "Vbg" {
        n618 = local read "Vbg array"() -> (w967:dbl[])
      }
      frame "Vtg" {
        n619 = local read "Vtg array"() -> (w968:dbl[])
      }
      frame "Ibg" {
        n620 = local read "Ibg array"() -> (w969:dbl[])
      }
      frame "Itg" {
        n621 = local read "Itg array"() -> (w970:dbl[])
      }
      frame "Vxx" {
        n622 = local read "Vxx array"() -> (w971:dbl[])
      }
      frame "Vxy" {
        n623 = local read "Vxy array"() -> (w972:dbl[])
      }
      frame "V/I 3" {
        n624 = local read "V/I3 array"() -> (w973:dbl[])
      }
      frame "V/I 4" {
        n625 = local read "V/I4 array"() -> (w974:dbl[])
      }
      frame "Rxy" {
        n626 = local read "Rxy Array"() -> (w975:dbl[])
      }
      frame "R2probe" {
        n627 = local read "R2probe array"() -> (w976:dbl[])
      }
      frame "Temperature" {
        n628 = local read "T"() -> (w977:dbl[])
      }
      frame "time" {
        n629 = local read "Time"() -> (w978:dbl[])
      }
      frame "V K2400_01" {
        n630 = local read "V K2400_01 array"() -> (w979:dbl[])
      }
      frame "V K2400_02" {
        n631 = local read "V K2400_02 array"() -> (w980:dbl[])
      }
      frame "I K2400_01" {
        n632 = local read "I K2400 01"() -> (w981:dbl[])
      }
      frame "I K2400_02" {
        n633 = local read "I K2400 02"() -> (w982:dbl[])
      }
      frame "DMM1".."DMM9" {
        n634 = Match Pattern(string=w990, regular expression="DMM") -> (after substring=w988:string)  [unwired: 1 in, 3 out]
        n635 = Scan Value(string=w988, format string="%g") -> (value=w985:dbl)  [unwired: 1 in, 1 out]
        n636 = local read "DMM Array"() -> (w986:dbl[][])
        n637 = Decrement(x=w985) -> (x-1=w983:dbl)
        n638 = Index Array(array=w986, index (col)=w983) -> (element=w984:dbl[])  [unwired: 1 in]
      }
      frame "X Lockin1".."X Lockin9" {
        n639 = Match Pattern(string=w998, regular expression="X Lockin") -> (after substring=w996:string)  [unwired: 1 in, 3 out]
        n640 = local read "Lockin X Array"() -> (w994:dbl[][])
        n641 = Scan Value(string=w996, format string="%g") -> (value=w993:dbl)  [unwired: 1 in, 1 out]
        n642 = Decrement(x=w993) -> (x-1=w991:dbl)
        n643 = Index Array(array=w994, index (col)=w991) -> (element=w992:dbl[])  [unwired: 1 in]
      }
      frame "Y Lockin1".."Y Lockin9" {
        n644 = Match Pattern(string=w1006, regular expression="Y Lockin") -> (after substring=w1004:string)  [unwired: 1 in, 3 out]
        n645 = local read "Lockin Y Array"() -> (w1002:dbl[][])
        n646 = Scan Value(string=w1004, format string="%g") -> (value=w1001:dbl)  [unwired: 1 in, 1 out]
        n647 = Decrement(x=w1001) -> (x-1=w999:dbl)
        n648 = Index Array(array=w1002, index (col)=w999) -> (element=w1000:dbl[])  [unwired: 1 in]
      }
      frame "Am Lockin1".."Am Lockin9" {
        n649 = local read "Lockin A Array"() -> (w1010:dbl[][])
        n650 = Match Pattern(string=w1014, regular expression="Am Lockin") -> (after substring=w1012:string)  [unwired: 1 in, 3 out]
        n651 = Scan Value(string=w1012, format string="%g") -> (value=w1009:dbl)  [unwired: 1 in, 1 out]
        n652 = Decrement(x=w1009) -> (x-1=w1007:dbl)
        n653 = Index Array(array=w1010, index (col)=w1007) -> (element=w1008:dbl[])  [unwired: 1 in]
      }
      frame "B" {
        n654 = local read "B"() -> (w1015:dbl[])
      }
      frame "R4probe" {
        n655 = local read "R4probe array"() -> (w1016:dbl[])
      }
      frame "Formula1" {
        n656 = local read "Formula1Array"() -> (w1017:dbl[])
      }
      frame "Formula2" {
        n657 = local read "Formula2Array"() -> (w1018:dbl[])
      }
      frame "Formula3" {
        n658 = local read "Formula3Array"() -> (w1019:dbl[])
      }
      frame "Formula4" {
        n659 = local read "Formula4Array"() -> (w1020:dbl[])
      }
    }
    n660 = case shown="\"Itg\"" "Y-Axis 2" {
      selector: "Y-Axis 2" -> [_ _ _ _ _ _ _ _ _ _ _ _ _ _ _ _ _ _ _ _ _ _ _ w929 w937 w945 w953 _ _ _ _ _ _]
      tunnel: [w899 w900 w901 w902 w903 w904 w905 w906 w907 w908 w909 w910 w911 w912 w913 w914 w915 w916 w917 w918 w919 w920 w921 w923 w931 w939 w947 w954 w955 w956 w957 w958 w959] -> w619
      frame "DAC 1 V", Default {
        n661 = local read "DAC 1 array"() -> (w899:dbl[])
      }
      frame "DAC 2 V" {
        n662 = local read "DAC 2 array"() -> (w900:dbl[])
      }
      frame "DAC 3 V" {
        n663 = local read "DAC 3 array"() -> (w901:dbl[])
      }
      frame "DAC 4 V" {
        n664 = local read "DAC 4 array"() -> (w902:dbl[])
      }
      frame "Wavelength" {
        n665 = local read "Wavelength array"() -> (w903:dbl[])
      }
      frame "Vsd" {
        n666 = local read "Vsd array"() -> (w904:dbl[])
      }
      frame "Isd" {
        n667 = local read "Isd array"() -> (w905:dbl[])
      }
      frame "Vbg" {
        n668 = local read "Vbg array"() -> (w906:dbl[])
      }
      frame "Vtg" {
        n669 = local read "Vtg array"() -> (w907:dbl[])
      }
      frame "Ibg" {
        n670 = local read "Ibg array"() -> (w908:dbl[])
      }
      frame "Itg" {
        n671 = local read "Itg array"() -> (w909:dbl[])
      }
      frame "Vxx" {
        n672 = local read "Vxx array"() -> (w910:dbl[])
      }
      frame "Vxy" {
        n673 = local read "Vxy array"() -> (w911:dbl[])
      }
      frame "V/I 3" {
        n674 = local read "V/I3 array"() -> (w912:dbl[])
      }
      frame "V/I 4" {
        n675 = local read "V/I4 array"() -> (w913:dbl[])
      }
      frame "Rxy" {
        n676 = local read "Rxy Array"() -> (w914:dbl[])
      }
      frame "R2probe" {
        n677 = local read "R2probe array"() -> (w915:dbl[])
      }
      frame "Temperature" {
        n678 = local read "T"() -> (w916:dbl[])
      }
      frame "time" {
        n679 = local read "Time"() -> (w917:dbl[])
      }
      frame "V K2400_01" {
        n680 = local read "V K2400_01 array"() -> (w918:dbl[])
      }
      frame "V K2400_02" {
        n681 = local read "V K2400_02 array"() -> (w919:dbl[])
      }
      frame "I K2400_01" {
        n682 = local read "I K2400 01"() -> (w920:dbl[])
      }
      frame "I K2400_02" {
        n683 = local read "I K2400 02"() -> (w921:dbl[])
      }
      frame "DMM1".."DMM9" {
        n684 = Match Pattern(string=w929, regular expression="DMM") -> (after substring=w927:string)  [unwired: 1 in, 3 out]
        n685 = Scan Value(string=w927, format string="%g") -> (value=w924:dbl)  [unwired: 1 in, 1 out]
        n686 = local read "DMM Array"() -> (w925:dbl[][])
        n687 = Decrement(x=w924) -> (x-1=w922:dbl)
        n688 = Index Array(array=w925, index (col)=w922) -> (element=w923:dbl[])  [unwired: 1 in]
      }
      frame "X Lockin1".."X Lockin9" {
        n689 = Match Pattern(string=w937, regular expression="X Lockin") -> (after substring=w935:string)  [unwired: 1 in, 3 out]
        n690 = local read "Lockin X Array"() -> (w933:dbl[][])
        n691 = Scan Value(string=w935, format string="%g") -> (value=w932:dbl)  [unwired: 1 in, 1 out]
        n692 = Decrement(x=w932) -> (x-1=w930:dbl)
        n693 = Index Array(array=w933, index (col)=w930) -> (element=w931:dbl[])  [unwired: 1 in]
      }
      frame "Y Lockin1".."Y Lockin9" {
        n694 = Match Pattern(string=w945, regular expression="Y Lockin") -> (after substring=w943:string)  [unwired: 1 in, 3 out]
        n695 = local read "Lockin Y Array"() -> (w941:dbl[][])
        n696 = Scan Value(string=w943, format string="%g") -> (value=w940:dbl)  [unwired: 1 in, 1 out]
        n697 = Decrement(x=w940) -> (x-1=w938:dbl)
        n698 = Index Array(array=w941, index (col)=w938) -> (element=w939:dbl[])  [unwired: 1 in]
      }
      frame "Am Lockin1".."Am Lockin9" {
        n699 = local read "Lockin A Array"() -> (w949:dbl[][])
        n700 = Match Pattern(string=w953, regular expression="Am Lockin") -> (after substring=w951:string)  [unwired: 1 in, 3 out]
        n701 = Scan Value(string=w951, format string="%g") -> (value=w948:dbl)  [unwired: 1 in, 1 out]
        n702 = Decrement(x=w948) -> (x-1=w946:dbl)
        n703 = Index Array(array=w949, index (col)=w946) -> (element=w947:dbl[])  [unwired: 1 in]
      }
      frame "B" {
        n704 = local read "B"() -> (w954:dbl[])
      }
      frame "R4probe" {
        n705 = local read "R4probe array"() -> (w955:dbl[])
      }
      frame "Formula1" {
        n706 = local read "Formula1Array"() -> (w956:dbl[])
      }
      frame "Formula2" {
        n707 = local read "Formula2Array"() -> (w957:dbl[])
      }
      frame "Formula3" {
        n708 = local read "Formula3Array"() -> (w958:dbl[])
      }
      frame "Formula4" {
        n709 = local read "Formula4Array"() -> (w959:dbl[])
      }
    }
    n710 = case shown="\"Itg\"" "X-Axis 1" {
      selector: "X-Axis 1" -> [_ _ _ _ _ _ _ _ _ _ _ _ _ _ _ _ _ _ _ _ _ _ _ w868 w876 w884 w892 _ _ _ _ _ _]
      tunnel: [w838 w839 w840 w841 w842 w843 w844 w845 w846 w847 w848 w849 w850 w851 w852 w853 w854 w855 w856 w857 w858 w859 w860 w862 w870 w878 w886 w893 w894 w895 w896 w897 w898] -> w617
      frame "DAC 1 V", Default {
        n711 = local read "DAC 1 array"() -> (w838:dbl[])
      }
      frame "DAC 2 V" {
        n712 = local read "DAC 2 array"() -> (w839:dbl[])
      }
      frame "DAC 3 V" {
        n713 = local read "DAC 3 array"() -> (w840:dbl[])
      }
      frame "DAC 4 V" {
        n714 = local read "DAC 4 array"() -> (w841:dbl[])
      }
      frame "Wavelength" {
        n715 = local read "Wavelength array"() -> (w842:dbl[])
      }
      frame "Vsd" {
        n716 = local read "Vsd array"() -> (w843:dbl[])
      }
      frame "Isd" {
        n717 = local read "Isd array"() -> (w844:dbl[])
      }
      frame "Vbg" {
        n718 = local read "Vbg array"() -> (w845:dbl[])
      }
      frame "Vtg" {
        n719 = local read "Vtg array"() -> (w846:dbl[])
      }
      frame "Ibg" {
        n720 = local read "Ibg array"() -> (w847:dbl[])
      }
      frame "Itg" {
        n721 = local read "Itg array"() -> (w848:dbl[])
      }
      frame "Vxx" {
        n722 = local read "Vxx array"() -> (w849:dbl[])
      }
      frame "Vxy" {
        n723 = local read "Vxy array"() -> (w850:dbl[])
      }
      frame "V/I 3" {
        n724 = local read "V/I3 array"() -> (w851:dbl[])
      }
      frame "V/I 4" {
        n725 = local read "V/I4 array"() -> (w852:dbl[])
      }
      frame "Rxy" {
        n726 = local read "Rxy Array"() -> (w853:dbl[])
      }
      frame "R2probe" {
        n727 = local read "R2probe array"() -> (w854:dbl[])
      }
      frame "Temperature" {
        n728 = local read "T"() -> (w855:dbl[])
      }
      frame "time" {
        n729 = local read "Time"() -> (w856:dbl[])
      }
      frame "V K2400_01" {
        n730 = local read "V K2400_01 array"() -> (w857:dbl[])
      }
      frame "V K2400_02" {
        n731 = local read "V K2400_02 array"() -> (w858:dbl[])
      }
      frame "I K2400_01" {
        n732 = local read "I K2400 01"() -> (w859:dbl[])
      }
      frame "I K2400_02" {
        n733 = local read "I K2400 02"() -> (w860:dbl[])
      }
      frame "DMM1".."DMM9" {
        n734 = Match Pattern(string=w868, regular expression="DMM") -> (after substring=w866:string)  [unwired: 1 in, 3 out]
        n735 = Scan Value(string=w866, format string="%g") -> (value=w863:dbl)  [unwired: 1 in, 1 out]
        n736 = local read "DMM Array"() -> (w864:dbl[][])
        n737 = Decrement(x=w863) -> (x-1=w861:dbl)
        n738 = Index Array(array=w864, index (col)=w861) -> (element=w862:dbl[])  [unwired: 1 in]
      }
      frame "X Lockin1".."X Lockin9" {
        n739 = Match Pattern(string=w876, regular expression="X Lockin") -> (after substring=w874:string)  [unwired: 1 in, 3 out]
        n740 = local read "Lockin X Array"() -> (w872:dbl[][])
        n741 = Scan Value(string=w874, format string="%g") -> (value=w871:dbl)  [unwired: 1 in, 1 out]
        n742 = Decrement(x=w871) -> (x-1=w869:dbl)
        n743 = Index Array(array=w872, index (col)=w869) -> (element=w870:dbl[])  [unwired: 1 in]
      }
      frame "Y Lockin1".."Y Lockin9" {
        n744 = Match Pattern(string=w884, regular expression="Y Lockin") -> (after substring=w882:string)  [unwired: 1 in, 3 out]
        n745 = local read "Lockin Y Array"() -> (w880:dbl[][])
        n746 = Scan Value(string=w882, format string="%g") -> (value=w879:dbl)  [unwired: 1 in, 1 out]
        n747 = Decrement(x=w879) -> (x-1=w877:dbl)
        n748 = Index Array(array=w880, index (col)=w877) -> (element=w878:dbl[])  [unwired: 1 in]
      }
      frame "Am Lockin1".."Am Lockin9" {
        n749 = local read "Lockin A Array"() -> (w888:dbl[][])
        n750 = Match Pattern(string=w892, regular expression="Am Lockin") -> (after substring=w890:string)  [unwired: 1 in, 3 out]
        n751 = Scan Value(string=w890, format string="%g") -> (value=w887:dbl)  [unwired: 1 in, 1 out]
        n752 = Decrement(x=w887) -> (x-1=w885:dbl)
        n753 = Index Array(array=w888, index (col)=w885) -> (element=w886:dbl[])  [unwired: 1 in]
      }
      frame "B" {
        n754 = local read "B"() -> (w893:dbl[])
      }
      frame "R4probe" {
        n755 = local read "R4probe array"() -> (w894:dbl[])
      }
      frame "Formula1" {
        n756 = local read "Formula1Array"() -> (w895:dbl[])
      }
      frame "Formula2" {
        n757 = local read "Formula2Array"() -> (w896:dbl[])
      }
      frame "Formula3" {
        n758 = local read "Formula3Array"() -> (w897:dbl[])
      }
      frame "Formula4" {
        n759 = local read "Formula4Array"() -> (w898:dbl[])
      }
    }
    n760 = case shown="\"Itg\"" "Y-Axis 1" {
      selector: "Y-Axis 1" -> [_ _ _ _ _ _ _ _ _ _ _ _ _ _ _ _ _ _ _ _ _ _ _ w807 w815 w823 w831 _ _ _ _ _ _]
      tunnel: [w777 w778 w779 w780 w781 w782 w783 w784 w785 w786 w787 w788 w789 w790 w791 w792 w793 w794 w795 w796 w797 w798 w799 w801 w809 w817 w825 w832 w833 w834 w835 w836 w837] -> w616
      frame "DAC 1 V", Default {
        n761 = local read "DAC 1 array"() -> (w777:dbl[])
      }
      frame "DAC 2 V" {
        n762 = local read "DAC 2 array"() -> (w778:dbl[])
      }
      frame "DAC 3 V" {
        n763 = local read "DAC 3 array"() -> (w779:dbl[])
      }
      frame "DAC 4 V" {
        n764 = local read "DAC 4 array"() -> (w780:dbl[])
      }
      frame "Wavelength" {
        n765 = local read "Wavelength array"() -> (w781:dbl[])
      }
      frame "Vsd" {
        n766 = local read "Vsd array"() -> (w782:dbl[])
      }
      frame "Isd" {
        n767 = local read "Isd array"() -> (w783:dbl[])
      }
      frame "Vbg" {
        n768 = local read "Vbg array"() -> (w784:dbl[])
      }
      frame "Vtg" {
        n769 = local read "Vtg array"() -> (w785:dbl[])
      }
      frame "Ibg" {
        n770 = local read "Ibg array"() -> (w786:dbl[])
      }
      frame "Itg" {
        n771 = local read "Itg array"() -> (w787:dbl[])
      }
      frame "Vxx" {
        n772 = local read "Vxx array"() -> (w788:dbl[])
      }
      frame "Vxy" {
        n773 = local read "Vxy array"() -> (w789:dbl[])
      }
      frame "V/I 3" {
        n774 = local read "V/I3 array"() -> (w790:dbl[])
      }
      frame "V/I 4" {
        n775 = local read "V/I4 array"() -> (w791:dbl[])
      }
      frame "Rxy" {
        n776 = local read "Rxy Array"() -> (w792:dbl[])
      }
      frame "R2probe" {
        n777 = local read "R2probe array"() -> (w793:dbl[])
      }
      frame "Temperature" {
        n778 = local read "T"() -> (w794:dbl[])
      }
      frame "time" {
        n779 = local read "Time"() -> (w795:dbl[])
      }
      frame "V K2400_01" {
        n780 = local read "V K2400_01 array"() -> (w796:dbl[])
      }
      frame "V K2400_02" {
        n781 = local read "V K2400_02 array"() -> (w797:dbl[])
      }
      frame "I K2400_01" {
        n782 = local read "I K2400 01"() -> (w798:dbl[])
      }
      frame "I K2400_02" {
        n783 = local read "I K2400 02"() -> (w799:dbl[])
      }
      frame "DMM1".."DMM9" {
        n784 = Match Pattern(string=w807, regular expression="DMM") -> (after substring=w805:string)  [unwired: 1 in, 3 out]
        n785 = Scan Value(string=w805, format string="%g") -> (value=w802:dbl)  [unwired: 1 in, 1 out]
        n786 = local read "DMM Array"() -> (w803:dbl[][])
        n787 = Decrement(x=w802) -> (x-1=w800:dbl)
        n788 = Index Array(array=w803, index (col)=w800) -> (element=w801:dbl[])  [unwired: 1 in]
      }
      frame "X Lockin1".."X Lockin9" {
        n789 = Match Pattern(string=w815, regular expression="X Lockin") -> (after substring=w813:string)  [unwired: 1 in, 3 out]
        n790 = local read "Lockin X Array"() -> (w811:dbl[][])
        n791 = Scan Value(string=w813, format string="%g") -> (value=w810:dbl)  [unwired: 1 in, 1 out]
        n792 = Decrement(x=w810) -> (x-1=w808:dbl)
        n793 = Index Array(array=w811, index (col)=w808) -> (element=w809:dbl[])  [unwired: 1 in]
      }
      frame "Y Lockin1".."Y Lockin9" {
        n794 = Match Pattern(string=w823, regular expression="Y Lockin") -> (after substring=w821:string)  [unwired: 1 in, 3 out]
        n795 = local read "Lockin Y Array"() -> (w819:dbl[][])
        n796 = Scan Value(string=w821, format string="%g") -> (value=w818:dbl)  [unwired: 1 in, 1 out]
        n797 = Decrement(x=w818) -> (x-1=w816:dbl)
        n798 = Index Array(array=w819, index (col)=w816) -> (element=w817:dbl[])  [unwired: 1 in]
      }
      frame "Am Lockin1".."Am Lockin9" {
        n799 = local read "Lockin A Array"() -> (w827:dbl[][])
        n800 = Match Pattern(string=w831, regular expression="Am Lockin") -> (after substring=w829:string)  [unwired: 1 in, 3 out]
        n801 = Scan Value(string=w829, format string="%g") -> (value=w826:dbl)  [unwired: 1 in, 1 out]
        n802 = Decrement(x=w826) -> (x-1=w824:dbl)
        n803 = Index Array(array=w827, index (col)=w824) -> (element=w825:dbl[])  [unwired: 1 in]
      }
      frame "B" {
        n804 = local read "B"() -> (w832:dbl[])
      }
      frame "R4probe" {
        n805 = local read "R4probe array"() -> (w833:dbl[])
      }
      frame "Formula1" {
        n806 = local read "Formula1Array"() -> (w834:dbl[])
      }
      frame "Formula2" {
        n807 = local read "Formula2Array"() -> (w835:dbl[])
      }
      frame "Formula3" {
        n808 = local read "Formula3Array"() -> (w836:dbl[])
      }
      frame "Formula4" {
        n809 = local read "Formula4Array"() -> (w837:dbl[])
      }
    }
    n810 = call "AxisLabel.vi"("Axis"="X-Axis 1") -> ("X Scale.Name Label.Text"=w647:string)
    n811 = call "AxisLabel.vi"("Axis"="Y-Axis 1") -> ("X Scale.Name Label.Text"=w646:string)
    n812 = local read "stopMainLoop"() -> (w653:bool)
    n813 = property on="Fig 2" class="XYGraph (strict)"("XScale.NameLbl.Text"=w649) -> ()  [unwired: 2 in, 2 out]
    n814 = Decimal String To Number(string="Fig3 Y scale") -> (number=w637:i32)  [unwired: 2 in, 1 out]
    n815 = Decimal String To Number(string="Fig4 Y scale") -> (number=w632:i32)  [unwired: 2 in, 1 out]
    n816 = Decimal String To Number(string="Fig2 Y scale") -> (number=w643:i32)  [unwired: 2 in, 1 out]
    n817 = Decimal String To Number(string="Fig1 Y scale") -> (number=w641:i32)  [unwired: 2 in, 1 out]
    n818 = call "AxisLabel.vi"("Axis"="X-Axis 4") -> ("X Scale.Name Label.Text"=w633:string)
    n819 = call "AxisLabel.vi"("Axis"="Y-Axis 4") -> ("X Scale.Name Label.Text"=w634:string)
    n820 = call "AxisLabel.vi"("Axis"="Y-Axis 2") -> ("X Scale.Name Label.Text"=w650:string)
    n821 = property on="Isd 3" class="XYGraph (strict)"("XScale.NameLbl.Text"=w639, "YScale.NameLbl.Text"=w638, "YScale.Mapping Mode"=w637) -> ()  [unwired: 2 in, 2 out]
    n822 = property on="Isd 4" class="XYGraph (strict)"("XScale.NameLbl.Text"=w633, "YScale.NameLbl.Text"=w634, "YScale.Mapping Mode"=w632) -> ()  [unwired: 2 in, 2 out]
    n823 = property on="Fig 2" class="XYGraph (strict)"("YScale.NameLbl.Text"=w650, "YScale.Mapping Mode"=w643) -> ()  [unwired: 2 in, 2 out]
    n824 = property on="Isd" class="XYGraph (strict)"("XScale.NameLbl.Text"=w647, "YScale.NameLbl.Text"=w646, "YScale.Mapping Mode"=w641) -> ()  [unwired: 2 in, 2 out]
    n825 = Quotient & Remainder(x=w631, y=2) -> (floor(x/y)=w629:i32)  [unwired: 1 out]
    n826 = event shown="[0] Timeout" {
      selector: _ -> [_ _ _ _ _]
      dyn-events: _ -> [_ _ _ _ _]
      timeout: w629 -> [_ _ _ _ _]
      tunnel: w652 -> [w1143 w1152 w1163 _ _]
      tunnel: [w1143 w1152 w1163 _ _] -> w651
      tunnel: w628 -> [_ _ _ w1165 w1183]
      tunnel: w627 -> [_ _ _ w1164 w1182]
      event Timeout {
        n827 = event-data() -> ()  [unwired: 1 in, 2 out]
      }
      event "Sensitivity Lockin1": Value Change {
        n828 = event-data() -> ()  [unwired: 1 in, 5 out]
        n829 = local read "LockinX"() -> (w1144:string[][])
        n830 = Index Array(array=w1144, index (row)=1 ("index")) -> (element=w1147:string[])  [unwired: 1 in]
        n831 = Concatenate Strings("GPIB0::" ("string"), w1147) -> (w1146:string)
        n832 = Type Cast(type=refnum<visa-resource-name> refnum ("VISA resource name"), x=w1146) -> (*(type *) &x=w1145:refnum<visa-resource-name>)
        n833 = call "Sr830sens_giulia.vi"("Sr 830 sensitivity"="Sensitivity Lockin1", "Change sensitivity ?"=TRUE, "SR830"=w1145) -> ()  [unwired: 1 out]
      }
      event "Sensitivity Lockin2": Value Change {
        n834 = event-data() -> ()  [unwired: 1 in, 5 out]
        n835 = local read "LockinX"() -> (w1155:string[][])
        n836 = Index Array(array=w1155, index (row)=1 ("index")) -> (element=w1157:string[])  [unwired: 1 in]
        n837 = Concatenate Strings("GPIB0::" ("string"), w1157) -> (w1156:string)
        n838 = Type Cast(type=refnum<visa-resource-name> refnum ("VISA resource name"), x=w1156) -> (*(type *) &x=w1154:refnum<visa-resource-name>)
        n839 = call "Sr830sens_giulia.vi"("Sr 830 sensitivity"="Sensitivity Lockin2", "Change sensitivity ?"=TRUE, "SR830"=w1154) -> ()  [unwired: 1 out]
      }
      event "DMMX": Value Change {
        n840 = event-data() -> ()  [unwired: 1 in, 5 out]
        n841 = local read "DMMX"() -> (w1168:string[][])
        n842 = Array Size(array=w1168) -> (size(s)=w1167:i32[])
        n843 = Index Array(array=w1167, index=0) -> (element=w1169:i32)
        n844 = for {
          N: w1169 -> [_]
          tunnel: w1168 -> [_] mode=indexing
          tunnel: [w1173] -> w1171 mode=indexing
          i -> [w1176]
          n845 = Increment(x=w1176) -> (x+1=w1174:i32)
          n846 = Number To Decimal String(number=w1174) -> (decimal integer string=w1175:string)  [unwired: 1 in]
          n847 = Concatenate Strings("DMM", w1175) -> (w1173:string)
        }
        n848 = Insert Into Array(array=w1164, new element=w1171) -> (w1172:string[])  [unwired: 1 in]
        n849 = Insert Into Array(array=w1165, new element=w1171) -> (w1170:string[])  [unwired: 1 in]
        n850 = property on="Vsd" class="CmbBox"("Strings[]"=w1172) -> ()  [unwired: 2 in, 2 out]
        n851 = property on="I leak BG" class="CmbBox"("Strings[]"=w1172) -> ()  [unwired: 2 in, 2 out]
        n852 = property on="I leak TG" class="CmbBox"("Strings[]"=w1172) -> ()  [unwired: 2 in, 2 out]
        n853 = property on="Vxx" class="CmbBox"("Strings[]"=w1172) -> ()  [unwired: 2 in, 2 out]
        n854 = property on="I 2probe 2" class="CmbBox"("Strings[]"=w1172) -> ()  [unwired: 2 in, 2 out]
        n855 = property on="Vxy" class="CmbBox"("Strings[]"=w1172) -> ()  [unwired: 2 in, 2 out]
        n856 = property on="V TG" class="CmbBox"("Strings[]"=w1172) -> ()  [unwired: 2 in, 2 out]
        n857 = property on="V BG" class="CmbBox"("Strings[]"=w1172) -> ()  [unwired: 2 in, 2 out]
        n858 = property on="Y-Axis 4" class="CmbBox"("Strings[]"=w1170) -> ()  [unwired: 2 in, 2 out]
        n859 = property on="X-Axis 4" class="CmbBox"("Strings[]"=w1170) -> ()  [unwired: 2 in, 2 out]
        n860 = property on="Y-Axis 1" class="CmbBox"("Strings[]"=w1170) -> ()  [unwired: 2 in, 2 out]
        n861 = property on="X-Axis 1" class="CmbBox"("Strings[]"=w1170) -> ()  [unwired: 2 in, 2 out]
        n862 = property on="X-Axis 2" class="CmbBox"("Strings[]"=w1170) -> ()  [unwired: 2 in, 2 out]
        n863 = property on="Y-Axis 2" class="CmbBox"("Strings[]"=w1170) -> ()  [unwired: 2 in, 2 out]
        n864 = property on="X-Axis 3" class="CmbBox"("Strings[]"=w1170) -> ()  [unwired: 2 in, 2 out]
        n865 = property on="Y-Axis 3" class="CmbBox"("Strings[]"=w1170) -> ()  [unwired: 2 in, 2 out]
      }
      event "LockinX": Value Change {
        n866 = event-data() -> ()  [unwired: 1 in, 5 out]
        n867 = local read "LockinX"() -> (w1181:string[][])
        n868 = Array Size(array=w1181) -> (size(s)=w1185:i32[])
        n869 = Index Array(array=w1185, index=0) -> (element=w1180:i32)
        n870 = for {
          N: w1180 -> [_]
          tunnel: w1181 -> [_] mode=indexing
          tunnel: [w1199] -> w1187 mode=indexing
          i -> [w1202]
          n871 = Increment(x=w1202) -> (x+1=w1200:i32)
          n872 = Number To Decimal String(number=w1200) -> (decimal integer string=w1201:string)  [unwired: 1 in]
          n873 = Concatenate Strings("DMM", w1201) -> (w1199:string)
        }
        n874 = for {
          N: w1180 -> [_]
          tunnel: [w1194] -> w1179 mode=indexing
          tunnel: w1181 -> [_] mode=indexing
          i -> [w1197]
          n875 = Increment(x=w1197) -> (x+1=w1195:i32)
          n876 = Number To Decimal String(number=w1195) -> (decimal integer string=w1196:string)  [unwired: 1 in]
          n877 = Concatenate Strings("Y Lockin", w1196) -> (w1194:string)
        }
        n878 = for {
          N: w1180 -> [_]
          tunnel: [w1189] -> w1178 mode=indexing
          tunnel: w1181 -> [_] mode=indexing
          i -> [w1192]
          n879 = Increment(x=w1192) -> (x+1=w1190:i32)
          n880 = Number To Decimal String(number=w1190) -> (decimal integer string=w1191:string)  [unwired: 1 in]
          n881 = Concatenate Strings("Am Lockin", w1191) -> (w1189:string)
        }
        n882 = Insert Into Array(array=w1183, new element #1=w1187, new element #2=w1179, new element #3=w1178) -> (w1186:string[])  [unwired: 1 in]
        n883 = Insert Into Array(array=w1182, new element #1=w1187, new element #2=w1179, new element #3=w1178) -> (w1188:string[])  [unwired: 1 in]
        n884 = property on="Y-Axis 4" class="CmbBox"("Strings[]"=w1186) -> ()  [unwired: 2 in, 2 out]
        n885 = property on="X-Axis 4" class="CmbBox"("Strings[]"=w1186) -> ()  [unwired: 2 in, 2 out]
        n886 = property on="Y-Axis 1" class="CmbBox"("Strings[]"=w1186) -> ()  [unwired: 2 in, 2 out]
        n887 = property on="X-Axis 1" class="CmbBox"("Strings[]"=w1186) -> ()  [unwired: 2 in, 2 out]
        n888 = property on="X-Axis 2" class="CmbBox"("Strings[]"=w1186) -> ()  [unwired: 2 in, 2 out]
        n889 = property on="Y-Axis 2" class="CmbBox"("Strings[]"=w1186) -> ()  [unwired: 2 in, 2 out]
        n890 = property on="X-Axis 3" class="CmbBox"("Strings[]"=w1186) -> ()  [unwired: 2 in, 2 out]
        n891 = property on="Y-Axis 3" class="CmbBox"("Strings[]"=w1186) -> ()  [unwired: 2 in, 2 out]
        n892 = property on="Vsd" class="CmbBox"("Strings[]"=w1188) -> ()  [unwired: 2 in, 2 out]
        n893 = property on="I leak BG" class="CmbBox"("Strings[]"=w1188) -> ()  [unwired: 2 in, 2 out]
        n894 = property on="I leak TG" class="CmbBox"("Strings[]"=w1188) -> ()  [unwired: 2 in, 2 out]
        n895 = property on="Vxx" class="CmbBox"("Strings[]"=w1188) -> ()  [unwired: 2 in, 2 out]
        n896 = property on="I 2probe 2" class="CmbBox"("Strings[]"=w1188) -> ()  [unwired: 2 in, 2 out]
        n897 = property on="Vxy" class="CmbBox"("Strings[]"=w1188) -> ()  [unwired: 2 in, 2 out]
        n898 = property on="V TG" class="CmbBox"("Strings[]"=w1188) -> ()  [unwired: 2 in, 2 out]
        n899 = property on="V BG" class="CmbBox"("Strings[]"=w1188) -> ()  [unwired: 2 in, 2 out]
      }
    }
    n900 = Bundle("Formula4Array"=w614, "Formula4Array"=w611) -> (→"Isd 3":T9)  [unwired: 1 out]
    n901 = Bundle("Formula4Array"=w625, "Formula4Array"=w623) -> (→"Isd 4":T9)  [unwired: 1 out]
    n902 = Bundle("Formula4Array"=w622, "Formula4Array"=w619) -> (→"Fig 2":T9)  [unwired: 1 out]
    n903 = Bundle("Formula4Array"=w617, "Formula4Array"=w616) -> (→"Isd":T9)  [unwired: 1 out]
  }
  n904 = Insert Into Array(array=w10, new element #1=w11, new element #2=w6, new element #3=w5) -> (w12:string[])  [unwired: 1 in]
  n905 = Insert Into Array(array=w9, new element #1=w11, new element #2=w6, new element #3=w5, new element #4=w2) -> (w1:string[])  [unwired: 1 in]
  n906 = property on="Y-Axis 4" class="CmbBox"("Strings[]"=w12) -> ()  [unwired: 2 in, 2 out]
  n907 = property on="X-Axis 4" class="CmbBox"("Strings[]"=w12) -> ()  [unwired: 2 in, 2 out]
  n908 = property on="Y-Axis 1" class="CmbBox"("Strings[]"=w12) -> ()  [unwired: 2 in, 2 out]
  n909 = property on="X-Axis 1" class="CmbBox"("Strings[]"=w12) -> ()  [unwired: 2 in, 2 out]
  n910 = property on="X-Axis 2" class="CmbBox"("Strings[]"=w12) -> ()  [unwired: 2 in, 2 out]
  n911 = property on="Y-Axis 2" class="CmbBox"("Strings[]"=w12) -> ()  [unwired: 2 in, 2 out]
  n912 = property on="X-Axis 3" class="CmbBox"("Strings[]"=w12) -> ()  [unwired: 2 in, 2 out]
  n913 = property on="Y-Axis 3" class="CmbBox"("Strings[]"=w12) -> ()  [unwired: 2 in, 2 out]
  n914 = property on="Vsd" class="CmbBox"("Strings[]"=w1) -> ()  [unwired: 2 in, 2 out]
  n915 = property on="I leak BG" class="CmbBox"("Strings[]"=w1) -> ()  [unwired: 2 in, 2 out]
  n916 = property on="I leak TG" class="CmbBox"("Strings[]"=w1) -> ()  [unwired: 2 in, 2 out]
  n917 = property on="Vxx" class="CmbBox"("Strings[]"=w1) -> ()  [unwired: 2 in, 2 out]
  n918 = property on="I 2probe 2" class="CmbBox"("Strings[]"=w1) -> ()  [unwired: 2 in, 2 out]
  n919 = property on="Vxy" class="CmbBox"("Strings[]"=w1) -> ()  [unwired: 2 in, 2 out]
  n920 = property on="V TG" class="CmbBox"("Strings[]"=w1) -> ()  [unwired: 2 in, 2 out]
  n921 = property on="V BG" class="CmbBox"("Strings[]"=w1) -> ()  [unwired: 2 in, 2 out]
  n922 = property on="V / I 3" class="CmbBox"("Strings[]"=w1) -> ()  [unwired: 2 in, 2 out]
  n923 = property on="V / I 4" class="CmbBox"("Strings[]"=w1) -> ()  [unwired: 2 in, 2 out]
